vi "Main.vi"(11 "Module Admin":refnum<class "Delacor_lib_QMH_Module Admin.lvclass">) -> ()   [LabVIEW 2019, in "Settings Editor.lvlib"]
doc: "This template is based off of the Queued Message Handler design pattern and the Queued Message Handler project template that ships with LabVIEW.\n\nThe main difference is that the queue is private to this module and communication between modules is performed via Broadcast and Request events.\n\nRequest events are wrapped in public API methods and are handled in the Event Handling Loop (EHL) of this VI. Any module can register for Broadcast events sent by this module. The EHL generates messages based on user interface actions.\n\nThe Message Handling Loop (MHL) processes messages generated by the EHL, or by other messages. The messages are string values, so new messages can be added easily to the Message Cases case structure in the MHL. Each message cluster can also provide an optional value for Message Data, which is a variant that can be converted to whatever message-specific data is required.\n_____\nBased on Delacor QMH Project Template 4.0.0.47.\n_____\nBased on DQMH Project Template 6.1.0.94.\n\n<b>Note:</b> This VI was modified by the <b>Validate DQMH Module</b> tool to add a call to the Error Reported VI at the end of the 'Exit' MHL frame."
uses:
  Settings Editor.lvlib
  <vilib>/Delacor/Delacor QMH/Libraries/Module Admin_class/Delacor_lib_QMH_Module Admin.lvclass
  Acquisition/Signal Type--enum.ctl
  Acquisition/Calibration Values--cluster.ctl
  CML Shared/EEG Channel Settings.ctl
  Module Data--cluster.ctl
  Settings--cluster.ctl
  Settings UI Controls.ctl
  Stop Argument--cluster.ctl
  <vilib>/Delacor/Delacor QMH/Libraries/Message Queue_class/Delacor_lib_QMH_Message Queue.lvclass/Delacor_lib_QMH_Message Queue.ctl
  Update Application Settings Argument--cluster.ctl
  Update Application Settings (Reply Payload)--cluster.ctl
  <vilib>/Delacor/Delacor QMH/Libraries/Module Admin_class/Delacor_lib_QMH_Module Admin.lvclass/Delacor_lib_QMH_Module Admin.ctl
  Set CNV Montage Argument--cluster.ctl
  Set Eyes OC Montage Argument--cluster.ctl
  <vilib>/Utility/sysdir.llb/System Directory Type.ctl
  <vilib>/Delacor/Delacor QMH/Libraries/Message Queue_class/Delacor_lib_QMH_Enqueue Message (Single).vi
  <vilib>/Delacor/Delacor QMH/Libraries/Module Admin_class/Delacor_lib_QMH_Get External Launch.vi
  <vilib>/Utility/error.llb/Error Cluster From Error Code.vi
  <vilib>/ErrorRing/Error Ring.xnode
  <vilib>/Delacor/Delacor QMH/Libraries/Message Queue_class/Delacor_lib_QMH_Message Queue.lvclass
  Acquisition/Acquisition.lvlib
  CML Shared/CML Shared.lvlib
  <vilib>/Utility/miscctls.llb/LVPointTypeDef.ctl
panel:
  in  "Settings.EEG Channels 3":T1={"16 EEG Channels"=[], "Gain"=24} {"16 EEG Channels"."Channel No" step=1}
  in  "Settings.EEG Channels 2":T1={"16 EEG Channels"=[], "Gain"=24} {"16 EEG Channels"."Channel No" step=1}
  in  "Settings Tab":enum32{"Main", "Montage Adder"}(tab)
  in  "Delete Montage":bool
  in  "LSL En enum":enum16{"LSL Disabled", "LSL Enabled"}(ring)
  in  "Log File Base Path":path
  in  "OK":bool
  in  "Cancel":bool
  in  "Soft Trig enum":T2(ring)
  in  "Montages":i32(listbox)
  in  "Add Montage":bool
  out "Name Ch 17":string="Fp1"
  out "En ch 17":bool=TRUE
  out "Ref ch 17":bool
  out "Ref ch 18":bool
  out "Name Ch 18":string="Fp2"
  out "En ch 18":bool=TRUE
  out "Ref ch 19":bool
  out "Name Ch 19":string="F3"
  out "En ch 19":bool=TRUE
  out "Name Ch 20":string="Fz"
  out "En ch 20":bool=TRUE
  out "Ref ch 20":bool
  out "Ref ch 21":bool
  out "Name Ch 21":string="F4"
  out "Ref ch 22":bool
  out "Name Ch 22":string="T3"
  out "Name Ch 23":string="C3"
  out "Ref ch 23":bool
  out "Ref ch 24":bool
  out "Name Ch 24":string="Cz"
  out "Ref ch 25":bool
  out "Name Ch 25":string="C4"
  out "Name Ch 26":string="T4"
  out "Ref ch 26":bool
  out "Ref ch 27":bool
  out "Name Ch 27":string="P3"
  out "Ref ch 28":bool
  out "Name Ch 28":string="Fz"
  out "Ref ch 29":bool
  out "Name Ch 29":string="P4"
  out "En ch 21":bool=TRUE
  out "Ref ch 30":bool
  out "Name Ch 30":string="O1"
  out "En ch 22":bool=TRUE
  out "Ref ch 31":bool
  out "Name Ch 31":string="O2"
  out "En ch 23":bool=TRUE
  out "Ref ch 32":bool=TRUE
  out "Name Ch 32":string="Ref"
  out "En ch 24":bool=TRUE
  out "En ch 25":bool=TRUE
  out "En ch 26":bool=TRUE
  out "En ch 27":bool=TRUE
  out "En ch 28":bool=TRUE
  out "En ch 29":bool=TRUE
  out "En ch 30":bool=TRUE
  out "En ch 31":bool=TRUE
  out "En ch 32":bool
  in  "En ALL":bool
  in  "Name Ch 1":string="Fp1"
  in  "En ch 1":bool=TRUE
  in  "Ref ch 1":bool
  in  "Ref ch 2":bool
  in  "Name Ch 2":string="Fp2"
  in  "En ch 2":bool=TRUE
  in  "Ref ch 3":bool
  in  "Name Ch 3":string="F3"
  in  "En ch 3":bool=TRUE
  in  "Name Ch 4":string="Fz"
  in  "En ch 4":bool=TRUE
  in  "Ref ch 4":bool
  in  "Ref ch 5":bool
  in  "Name Ch 5":string="F4"
  in  "Ref ch 6":bool
  in  "Name Ch 6":string="T3"
  in  "Name Ch 7":string="C3"
  in  "Ref ch 7":bool
  in  "Ref ch 8":bool
  in  "Name Ch 8":string="Cz"
  in  "Ref ch 9":bool
  in  "Name Ch 9":string="C4"
  in  "Name Ch 10":string="T4"
  in  "Ref ch 10":bool
  in  "Ref ch 11":bool
  in  "Name Ch 11":string="P3"
  in  "Ref ch 12":bool
  in  "Name Ch 12":string="Fz"
  in  "Ref ch 13":bool
  in  "Name Ch 13":string="P4"
  in  "En ch 13":bool=TRUE
  in  "Ref ch 14":bool
  in  "Name Ch 14":string="O1"
  in  "En ch 14":bool=TRUE
  in  "Ref ch 15":bool
  in  "Name Ch 15":string="O2"
  in  "En ch 15":bool=TRUE
  in  "Ref ch 16":bool=TRUE
  in  "Name Ch 16":string="Ref"
  in  "En ch 16":bool=TRUE
  in  "En ch 5":bool=TRUE
  in  "En ch 6":bool=TRUE
  in  "En ch 7":bool=TRUE
  in  "En ch 8":bool=TRUE
  in  "En ch 9":bool=TRUE
  in  "En ch 10":bool=TRUE
  in  "En ch 11":bool=TRUE
  in  "En ch 12":bool
  in  "New Montage Name":string
  in  "Save Montage Button":bool
  in  "Cancel Save":bool
  in  "Settings.EEG Channels":T1={"16 EEG Channels"=[], "Gain"=24} {"16 EEG Channels"."Channel No" step=1}
  in  "Calibration Values":T3[](array[typedef])
  in  "Signal Type":T4
  out "error out":errorcluster
  # "Channel 1"
  # "Channel 2"
  # "Channel 3"
  # "Channel 4"
  # "Channel 5"
  # "Channel 6"
  # "Channel 7"
  # "Channel 8"
  # "Channel 9"
  # "Channel 10"
  # "Soft Trigger Settings"
  # "Channel 11"
  # "Channel 12"
  # "LSL Settings"
  # "Channel 13"
  # "Channel 14"
  # "Channel 15"
  # "Channel 16"
  # "Channel 1"
  # "Channel 2"
  # "Channel 3"
  # "Channel 4"
  # "Channel 5"
  # "Channel 6"
  # "Channel 7"
  # "Channel 8"
  # "Channel 9"
  # "Channel 10"
  # "Channel 11"
  # "Channel 12"
  # "Channel 13"
  # "Channel 14"
  # "Channel 15"
  # "Channel 16"
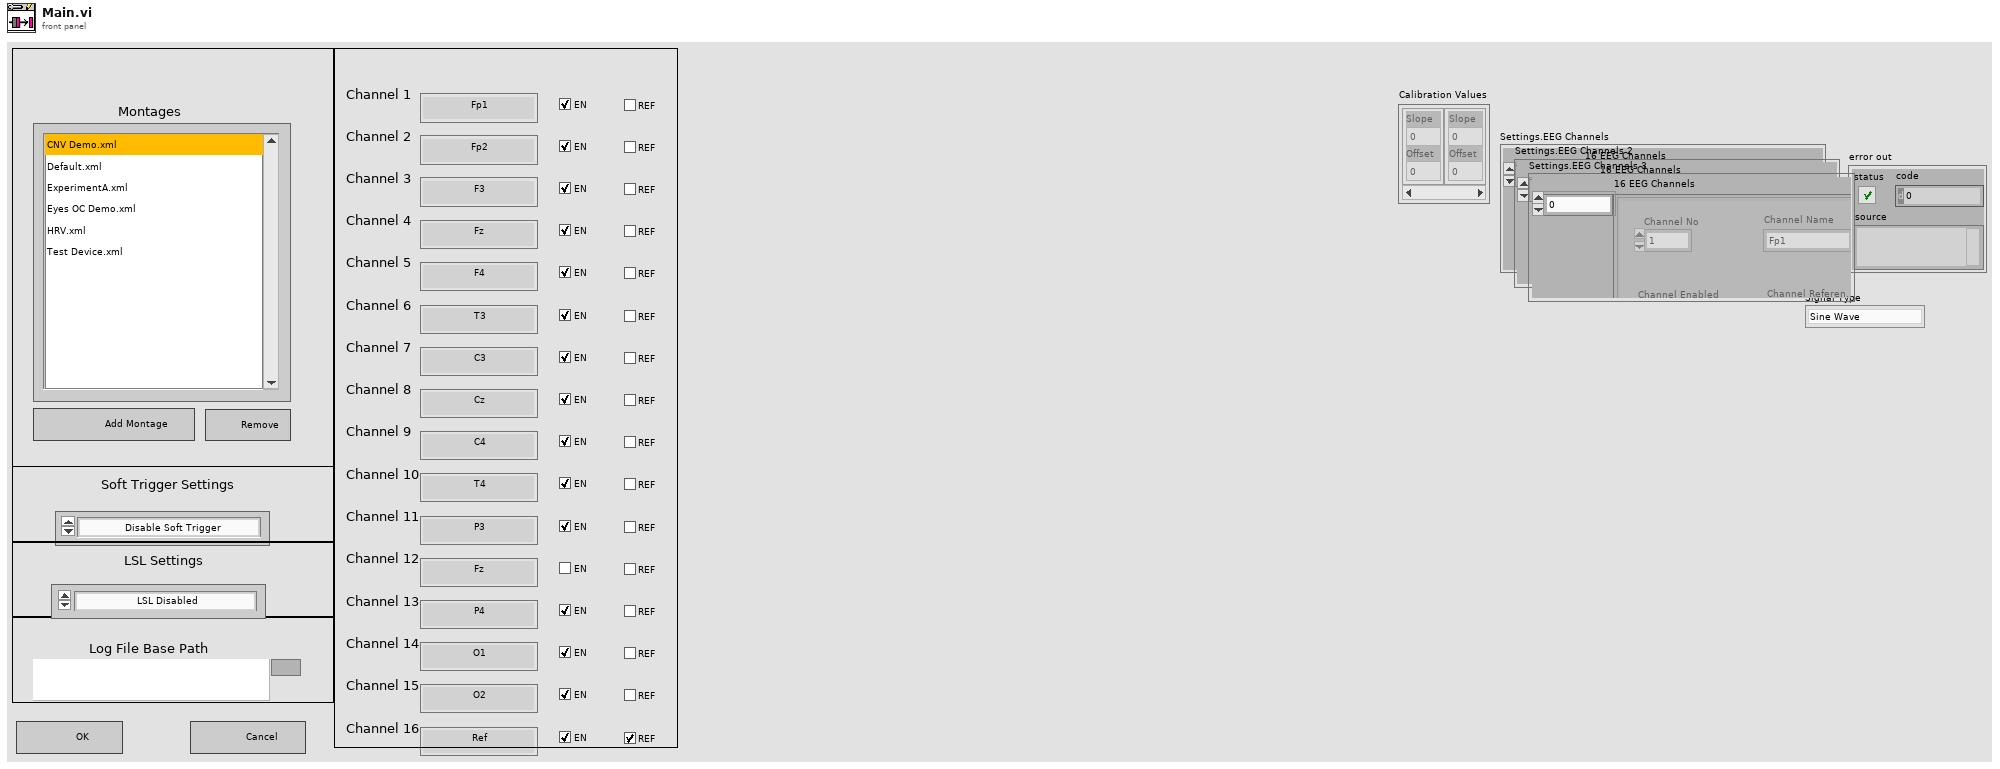
[diagram p1: front panel]
types:
  T1 = typedef "CML Shared.lvlib/EEG Channel Settings.ctl" = cluster{"16 EEG Channels":cluster{"Channel Name":string, "Channel No":u8, "Channel Enabled":bool, "Channel Referenced":bool}[], "Gain":u8}
  T2 = enum16{"Disable Soft Trigger", "Enable Soft Trigger"}
  T3 = typedef "Acquisition.lvlib/Calibration Values--cluster.ctl" = cluster{"Slope":dbl, "Offset":dbl}
  T4 = typedef "Acquisition.lvlib/Signal Type--enum.ctl" = enum16{"Sine Wave", "Square with Noise"}
  T5 = typedef "Settings Editor.lvlib/Request Events--cluster.ctl" = cluster{"Stop Module":refnum<user-event>, "Show Panel":refnum<user-event>, "Hide Panel":refnum<user-event>, "Get Module Execution Status":refnum<user-event>, "Show Diagram":refnum<user-event>, "Update Application Settings":refnum<user-event>, "Set CNV Montage":refnum<user-event>, "Set Eyes OC Montage":refnum<user-event>}
  T6 = typedef "Settings Editor.lvlib/Module Data--cluster.ctl" = cluster{"Settings":T7, "Settings Tab":refnum<vi>, "Controls UI":T8}
  T7 = typedef "Settings Editor.lvlib/Settings--cluster.ctl" = cluster{"Signal Type":T4, "Calibration Array":T3[], "Log File Base Path":path, "EEG Channels":T1, "Soft Trig enum":enum16{"Disable Soft Trigger", "Enable Soft Trigger"}, "Montage selection":cluster{"Montages Ref":refnum<vi>, "Selected Montage Number":u8, "Montages Names":string[]}, "LSL En enum":enum16{"LSL Disabled", "LSL Enabled"}}
  T8 = typedef "Settings Editor.lvlib/Settings UI Controls.ctl" = cluster{"En ch 1":refnum<vi>, "En ch 2":refnum<vi>, "En ch 3":refnum<vi>, "En ch 4":refnum<vi>, "En ch 5":refnum<vi>, "En ch 6":refnum<vi>, "En ch 7":refnum<vi>, "En ch 8":refnum<vi>, "En ch 9":refnum<vi>, "En ch 10":refnum<vi>, "En ch 11":refnum<vi>, "En ch 12":refnum<vi>, "En ch 13":refnum<vi>, "En ch 14":refnum<vi>, "En ch 15":refnum<vi>, "En ch 16":refnum<vi>, "Delete Montage":refnum<vi>}
  T9 = enum32{"invalid lock state", "Not Locked", "Locked (No Password)", "Password-protected"}
  T10 = typedef "Settings Editor.lvlib/Stop Argument--cluster.ctl" = cluster{"Origin":string, "Exit via Stop Module Req?":bool, "Wait for Module to stop?":bool}
  T11 = typedef "Settings Editor.lvlib/Update Application Settings Argument--cluster.ctl" = cluster{"Wait Notifier":refnum<notifier>, "wait for reply":bool}
  T12 = typedef "Settings Editor.lvlib/Set CNV Montage Argument--cluster.ctl" = cluster{"Boolean":bool}
  T13 = typedef "Settings Editor.lvlib/Set Eyes OC Montage Argument--cluster.ctl" = cluster{"Boolean":bool}
  T14 = enum32{"Invalid", "Standard", "Closed", "Hidden", "Minimized", "Maximized"}
  T15 = typedef "LVPointTypeDef.ctl" = cluster{"Horizontal":i16, "Vertical":i16}
  T16 = typedef "Settings Editor.lvlib/Update Application Settings (Reply Payload)--cluster.ctl" = cluster{"Settings":T7, "error":errorcluster}
  T17 = typedef "System Directory Type.ctl" = i32
  T18 = cluster{"Channel Name":string, "Channel No":u8, "Channel Enabled":bool, "Channel Referenced":bool}[]
  T19 = cluster{"Channel Name":string, "Channel No":u8, "Channel Enabled":bool, "Channel Referenced":bool}
  T20 = cluster{"Montages Ref":refnum<vi>, "Selected Montage Number":u8, "Montages Names":string[]}
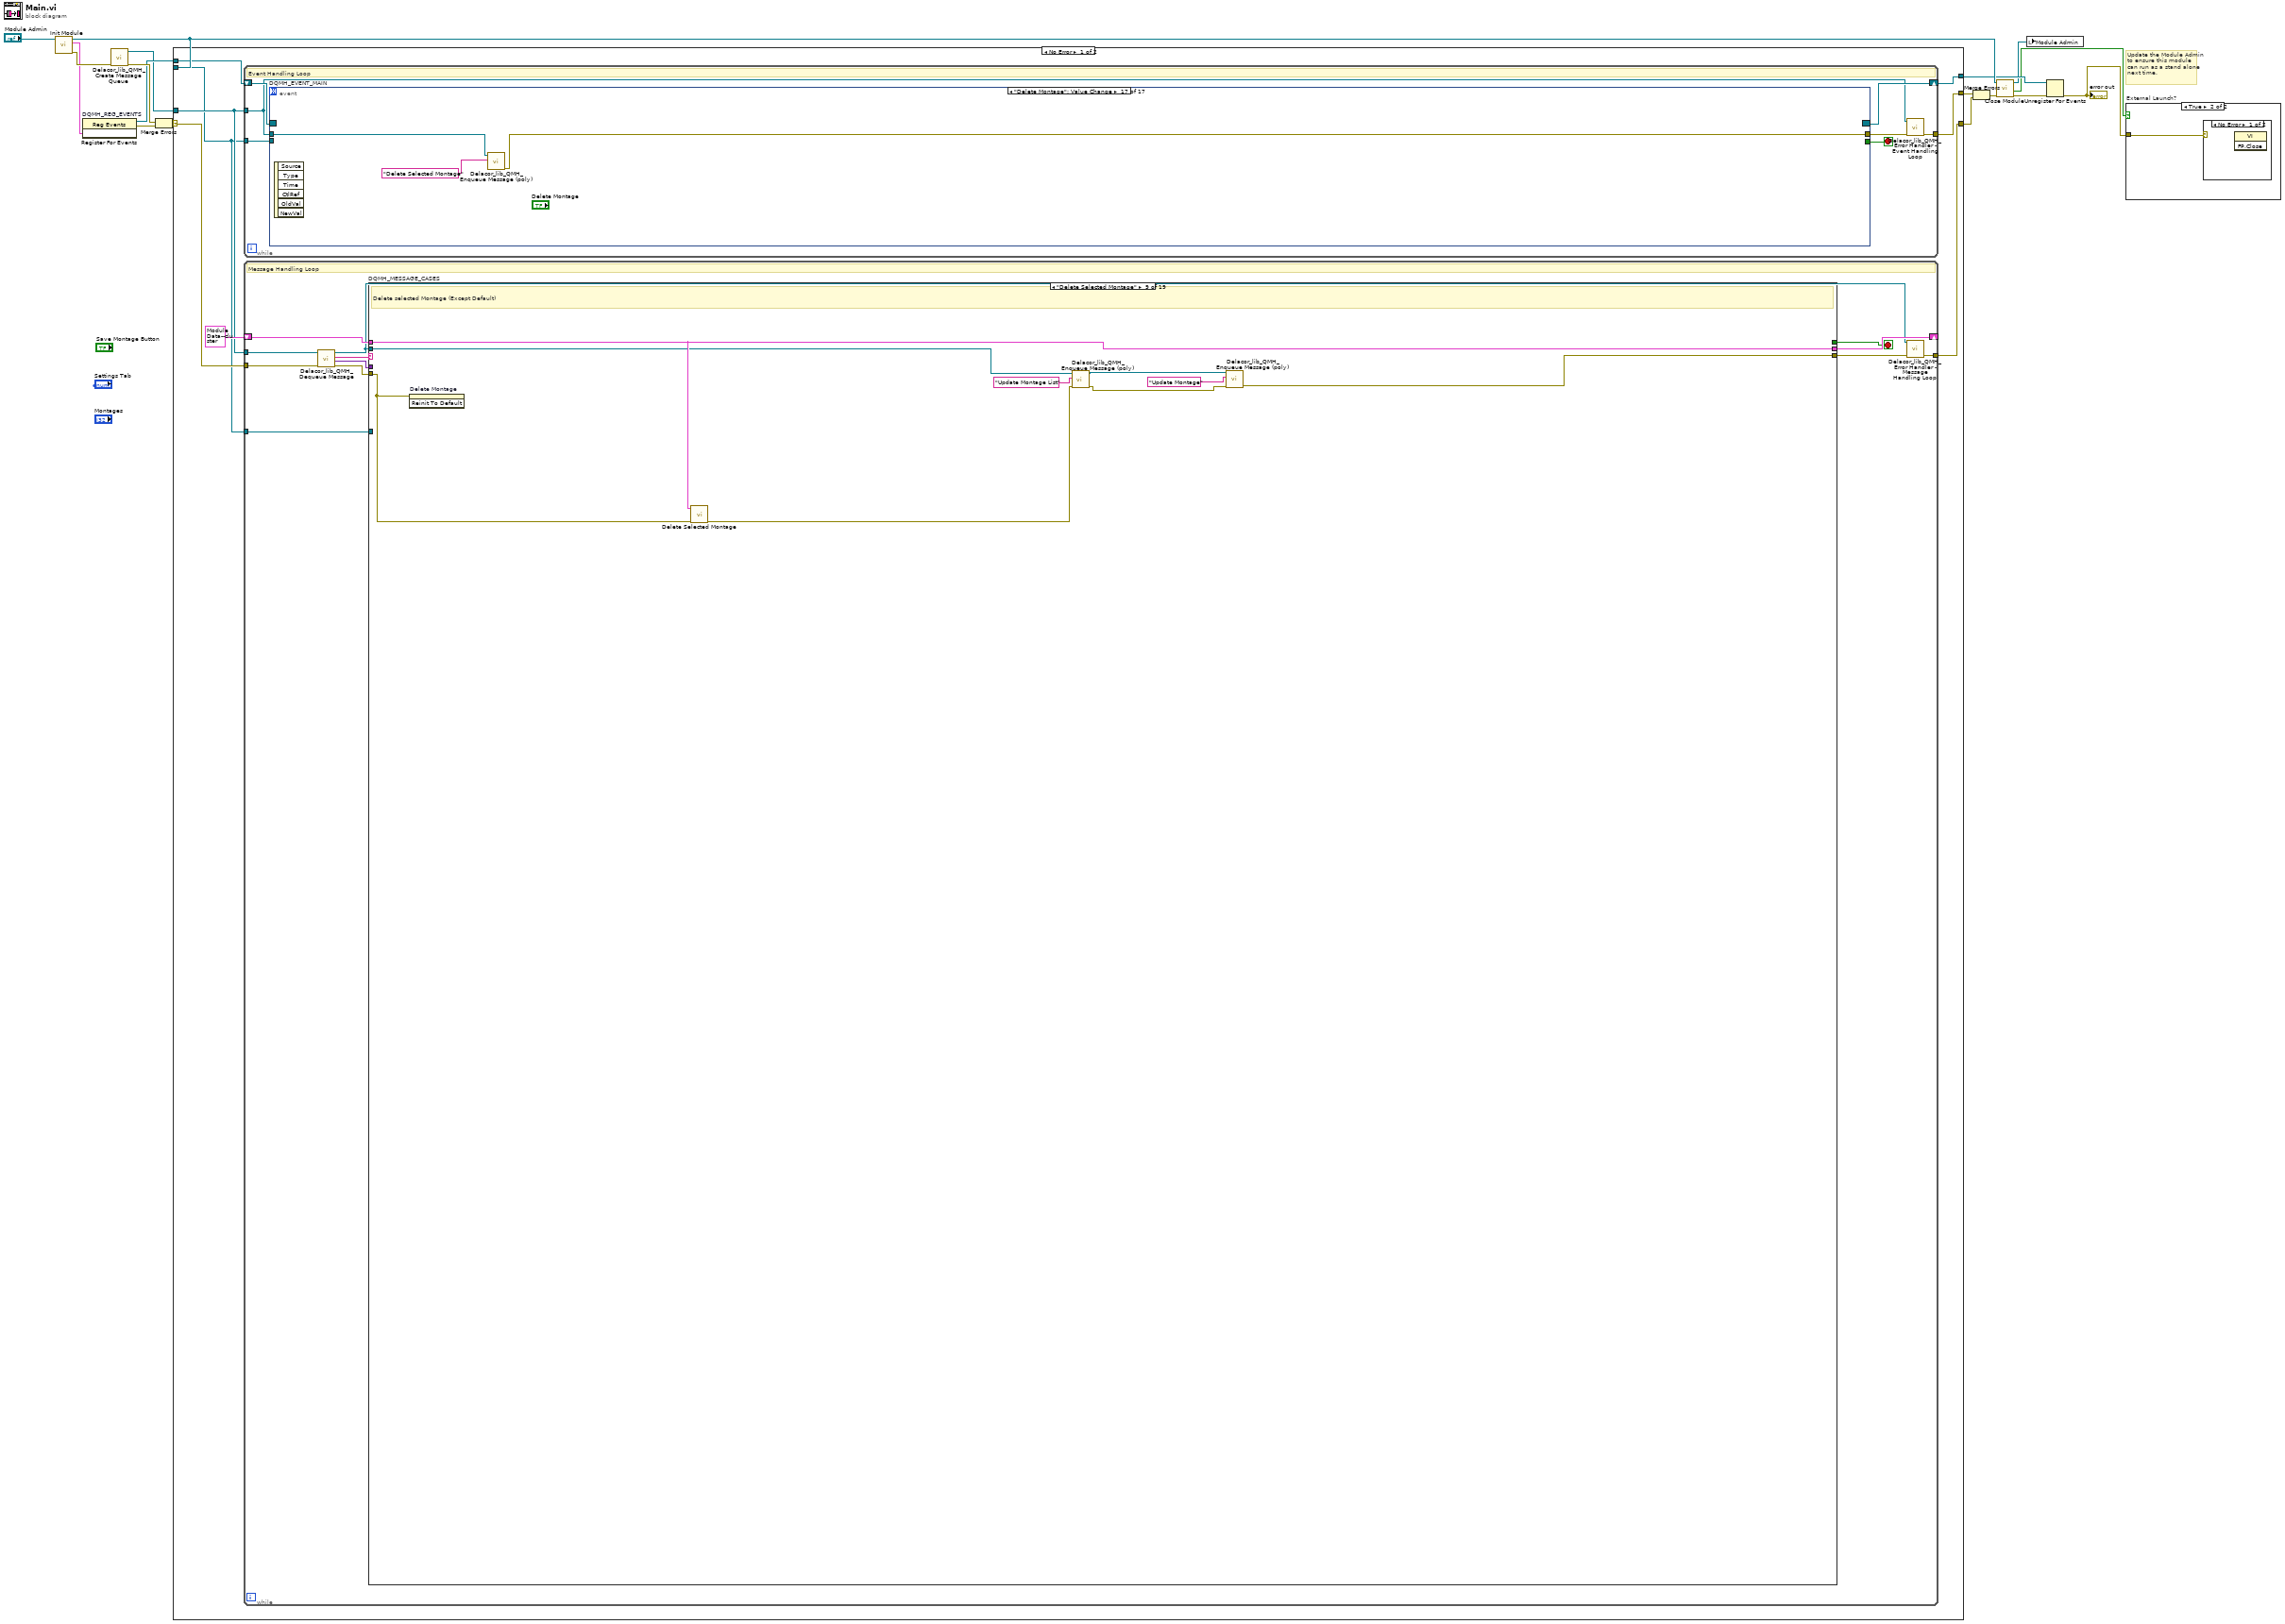
[diagram p0: block diagram]
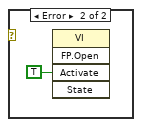
[diagram p3: hidden frame]
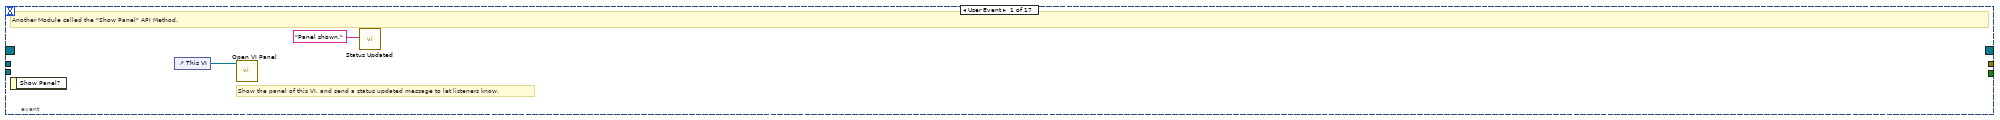
[diagram p4: hidden frame]
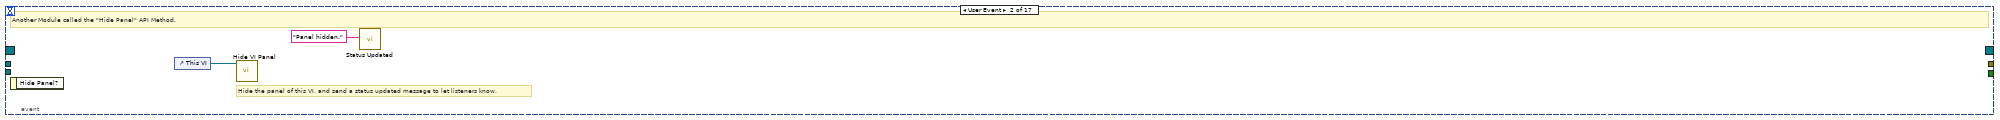
[diagram p5: hidden frame]
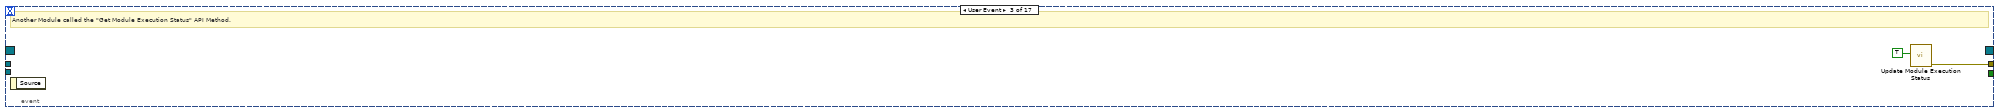
[diagram p6: hidden frame]
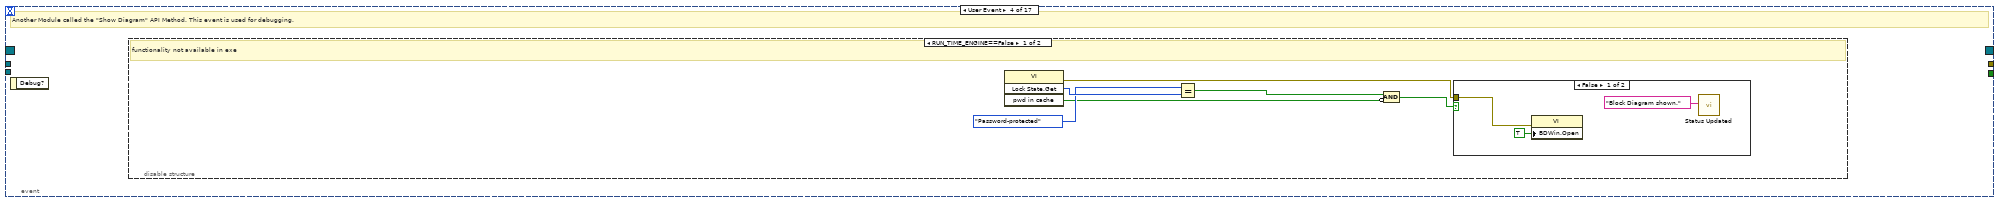
[diagram p7: hidden frame]
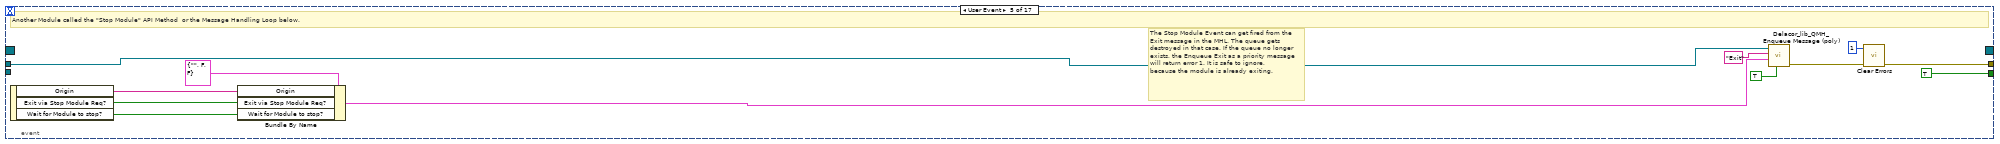
[diagram p10: hidden frame]
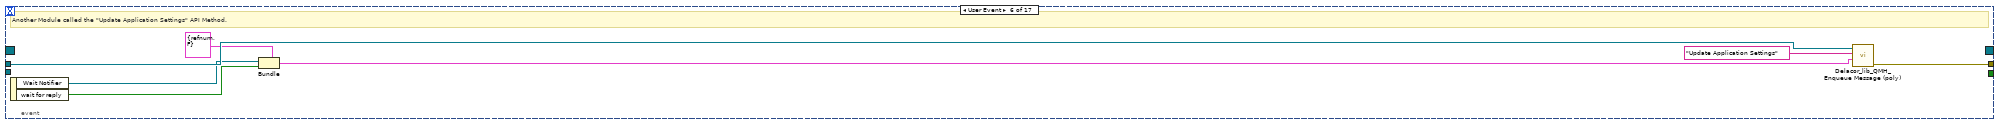
[diagram p11: hidden frame]
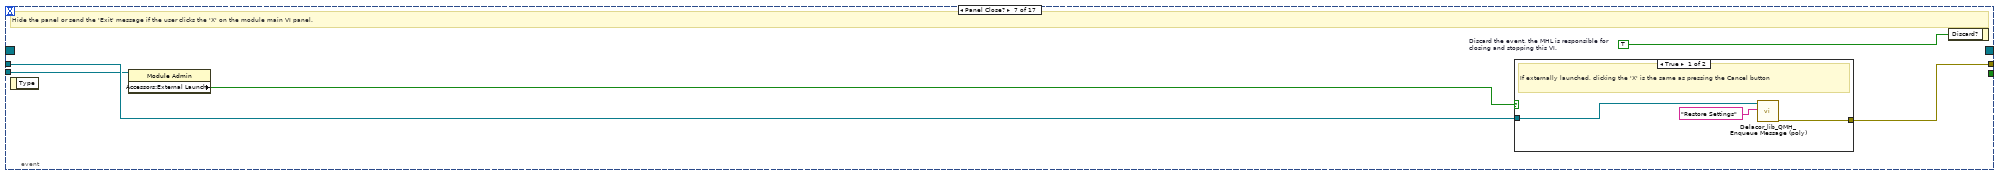
[diagram p12: hidden frame]
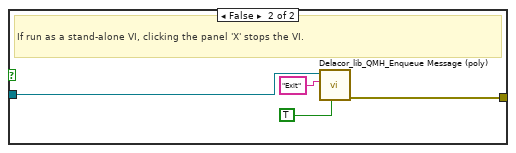
[diagram p13: hidden frame]
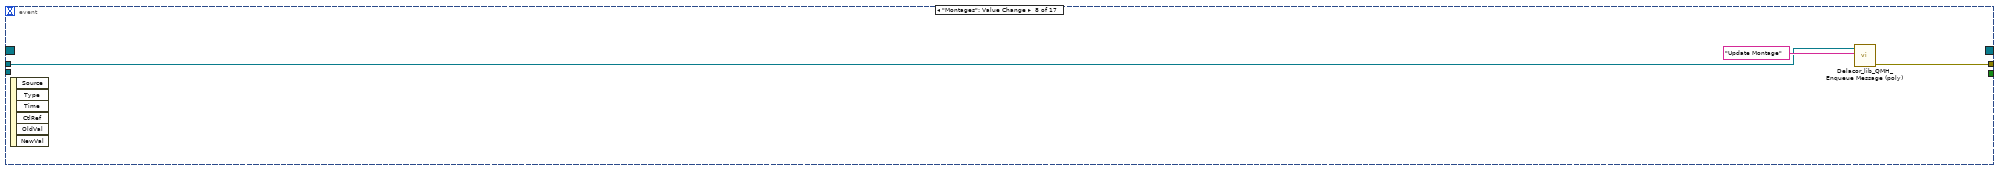
[diagram p14: hidden frame]
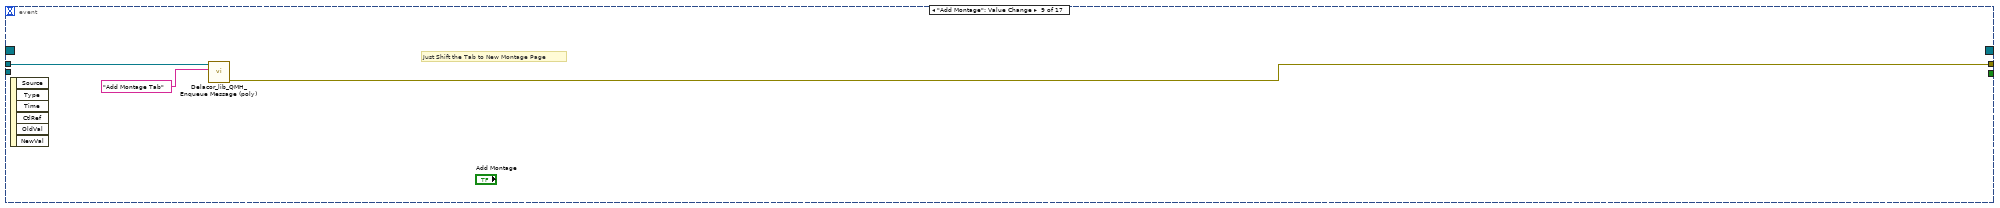
[diagram p15: hidden frame]
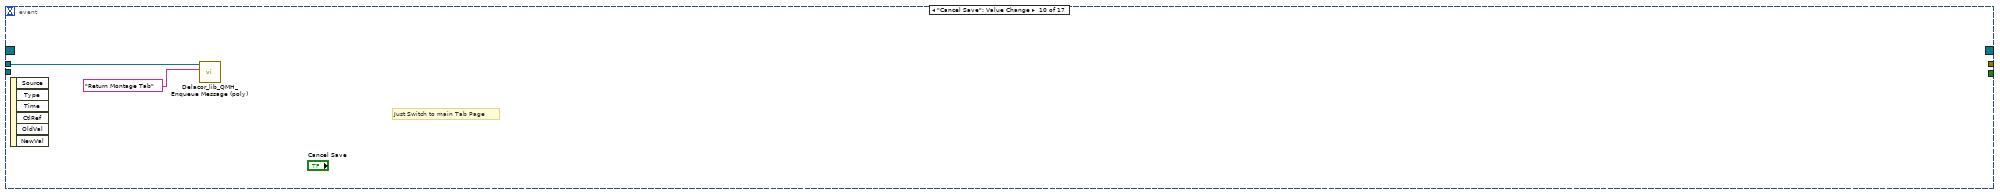
[diagram p16: hidden frame]
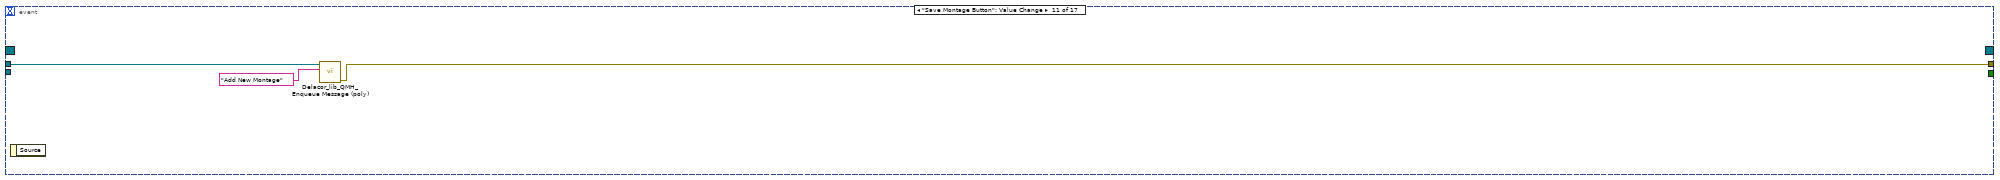
[diagram p17: hidden frame]
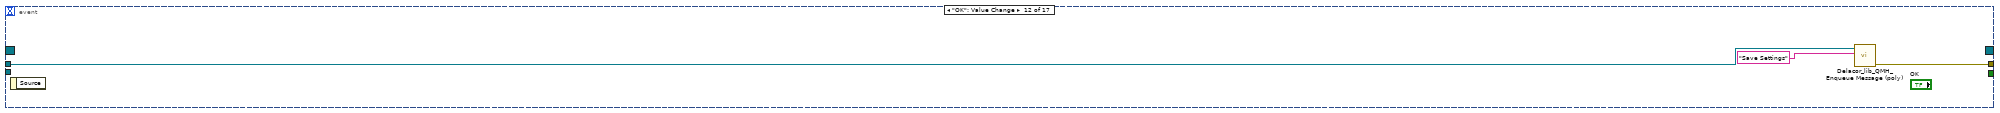
[diagram p18: hidden frame]
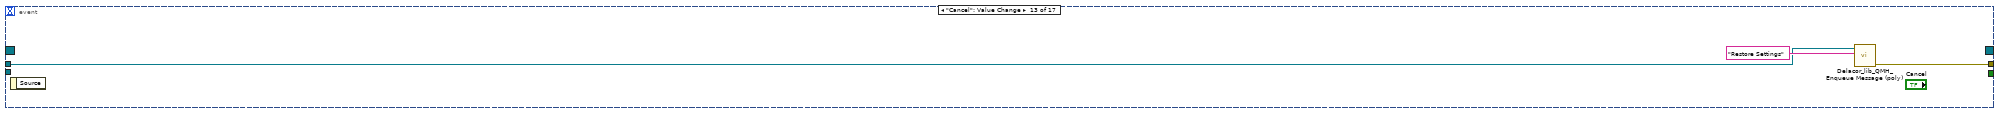
[diagram p19: hidden frame]
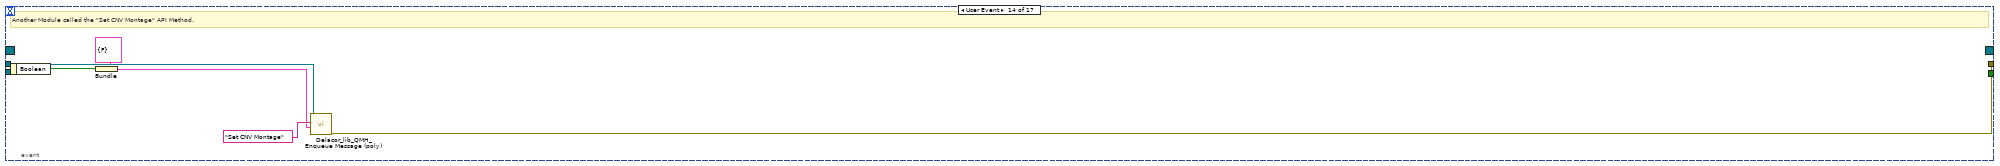
[diagram p20: hidden frame]
diagram:
  # "Update the Module Admin to ensure this module can run as a stand alone next time."
  n1 = call "Init Module.vi"("Singleton Module Admin in"="Module Admin") -> ("error out"=w16:errorcluster, "Settings Editor Request Events"=w5:T5, "Singleton Module Admin out"=w8:refnum<class "Delacor_lib_QMH_Module Admin.lvclass">)  [unwired: 8 in]
  n2 = register-events "DQMH_REG_EVENTS"(w5) -> (reference out=w6:refnum<event-registration>, error out=w9:errorcluster)  [unwired: 2 in]
  n3 = call <vilib>:"Delacor_lib_QMH_Create Message Queue.vi"("error in"=w16) -> ("error out"=w11:errorcluster, "Message Queue"=w4:refnum<class "Delacor_lib_QMH_Message Queue.lvclass">)  [unwired: 9 in]
  n4 = Merge Errors(w11, w9) -> (w10:errorcluster)
  n5 = case shown="No Error" w10 {
    selector: w10 -> [w23 w909]
    tunnel: [w25 w908] -> w17
    tunnel: [w22 w915] -> w7
    tunnel: w6 -> [w20 w915]
    tunnel: w4 -> [w19 w910]
    tunnel: [w24 _] -> w14
    tunnel: w8 -> [w18 w911]
    frame No Error {
      n6 = while {
        tunnel: w19 -> [w26]
        shift-right: [w29] -> w22
        shift-left: w20 -> [w30]
        tunnel: [w31] -> w24
        tunnel: w18 -> [w27]
        stop <- w28 stop-if-true
        # "Event Handling Loop"
        n7 = event "DQMH_EVENT_MAIN" shown="[16] \"Delete Montage\": Value Change" {
          selector: w30 -> [_ _ _ _ _ _ _ _ _ _ _ _ _ _ _ _ _]
          dyn-events: [_ _ _ _ _ _ _ _ _ _ _ _ _ _ _ _ _] -> w29
          timeout: _ -> [_ _ _ _ _ _ _ _ _ _ _ _ _ _ _ _ _]
          tunnel: [_ _ _ _ TRUE ("Discard?") _ _ _ _ _ _ _ _ _ _ _ _] -> w28
          tunnel: w26 -> [_ _ _ _ w55 w66 w69 w80 w83 w85 w88 w90 w94 w101 w107 w110 w113]
          tunnel: [_ _ w38 _ w58 w62 w71 w79 w82 _ w87 w91 w93 w96 w102 w108 w112] -> w32
          tunnel: w27 -> [_ _ _ _ _ _ w68 _ _ _ _ _ _ _ _ _ _]
          event User Event {
            # "Show the panel of this VI, and send a status updated message to let listeners know."
            # "Another Module called the \"Show Panel\" API Method."
            n8 = event-data() -> ()  [unwired: 1 in, 1 out]
            n9 = control-ref of="This VI"() -> (w34:refnum<vi>)
            n10 = call "Open VI Panel.vi"("VI"=w34) -> ()  [unwired: 10 in, 1 out]
            n11 = call "Status Updated.vi"("Status"="Panel shown." ("format string")) -> ()  [unwired: 10 in, 1 out]
          }
          event User Event {
            # "Hide the panel of this VI, and send a status updated message to let listeners know."
            # "Another Module called the \"Hide Panel\" API Method."
            n12 = event-data() -> ()  [unwired: 1 in, 1 out]
            n13 = control-ref of="This VI"() -> (w36:refnum<vi>)
            n14 = call "Hide VI Panel.vi"("VI"=w36) -> ()  [unwired: 10 in, 1 out]
            n15 = call "Status Updated.vi"("Status"="Panel hidden." ("format string")) -> ()  [unwired: 10 in, 1 out]
          }
          event User Event {
            # "Another Module called the \"Get Module Execution Status\" API Method."
            n16 = event-data() -> ()  [unwired: 1 in, 1 out]
            n17 = call "Update Module Execution Status.vi"("Running?"=TRUE) -> ("error out"=w38:errorcluster)  [unwired: 10 in]
          }
          event User Event {
            # "Another Module called the \"Show Diagram\" API Method. This event is used for debugging."
            n18 = event-data() -> ()  [unwired: 1 in, 1 out]
            n19 = disable-structure shown="RUN_TIME_ENGINE==False" {
              frame condition #0 (active) {
                # "functionality not available in exe"
                n20 = invoke class="VI" method="Lock State.Get"() -> (error out=w44:errorcluster, "Get Lock State"=w43:T9, "pwd in cache"=w40:bool)  [unwired: 4 in, 1 out]
                n21 = Equal?(x=T9."Password-protected", y=w43) -> (x = y?=w41:bool)
                n22 = Compound Arithmetic op=AND(w41, invert w40) -> (w39:bool)
                n23 = case shown="False" w39 {
                  tunnel: w44 -> [w47 _]
                  frame False {
                    n24 = property class="VI"(error in=w47, "BDWin.Open"=TRUE ("Block Diagram Window:Open")) -> ()  [unwired: 1 in, 2 out]
                    n25 = call "Status Updated.vi"("Status"="Block Diagram shown." ("format string")) -> ()  [unwired: 10 in, 1 out]
                  }
                  frame True {
                    # "Password-protected VI, and the password is not in the cache. Do not show the diagram."
                  }
                }
              }
              frame condition #1 {
              }
            }
          }
          event User Event {
            # "The Stop Module Event can get fired from the Exit message in the MHL. The queue gets destroyed in that case. If the queue no longer exists, the Enqueue Exit as a priority message will return error 1. It is safe to ignore, because the module is already exiting."
            # "Another Module called the \"Stop Module\" API Method  or the Message Handling Loop below."
            n26 = event-data() -> ("Origin"=w48:string, "Exit via Stop Module Req?"=w51:bool, "Wait for Module to stop?"=w50:bool)  [unwired: 1 in]
            n27 = Bundle By Name(cluster=T10 {"Origin"="", "Exit via Stop Module Req?"=FALSE, "Wait for Module to stop?"=FALSE} ("Stop Argument"), "Origin"=w48, "Exit via Stop Module Req?"=w51, "Wait for Module to stop?"=w50) -> (w49:T10)
            n28 = call-poly <vilib>:"Delacor_lib_QMH_Enqueue Message (poly).vi"("Priority Message? (F)"=TRUE, "Message Data"=w49, "Message"="Exit", "Message Queue in"=w55) -> ("error out"=w59:errorcluster)  [unwired: 6 in, 1 out]
            n29 = call <vilib>:"Clear Errors.vi"("error in (no error)"=w59, "specific error code to clear (0: all)"=1) -> ("error out"=w58:errorcluster)  [unwired: 4 in, 1 out]
          }
          event User Event {
            # "Another Module called the \"Update Application Settings\" API Method."
            n30 = event-data() -> ("Wait Notifier"=w61:refnum<notifier>, "wait for reply"=w60:bool)  [unwired: 1 in]
            n31 = Bundle(cluster=T11 {"Wait Notifier"=refnum, "wait for reply"=FALSE} ("Update Application Settings Argument"), "Wait Notifier"=w61, "wait for reply"=w60) -> (w63:T11)
            n32 = call-poly <vilib>:"Delacor_lib_QMH_Enqueue Message (poly).vi"("Message Data"=w63, "Message"="Update Application Settings", "Message Queue in"=w66) -> ("error out"=w62:errorcluster)  [unwired: 7 in, 1 out]
          }
          event Panel Close? {
            w70 = TRUE  # Discard the event, the MHL is responsible for closing and stopping this VI.
            # "Hide the panel or send the 'Exit' message if the user clicks the 'X' on the module main VI panel."
            n33 = event-data() -> ()  [unwired: 1 in, 1 out]
            n34 = property class="Module Admin"(reference=w68) -> ("Accessors:External Launch"=w67:bool)  [unwired: 1 in, 2 out]
            n35 = case shown="True" w67 {
              tunnel: w69 -> [w73 w77]
              tunnel: [w72 w78] -> w71
              frame True {
                # "If externally launched, clicking the 'X' is the same as pressing the Cancel button"
                n36 = call-poly <vilib>:"Delacor_lib_QMH_Enqueue Message (poly).vi"("Message"="Restore Settings", "Message Queue in"=w73) -> ("error out"=w72:errorcluster)  [unwired: 8 in, 1 out]
              }
              frame False {
                # "If run as a stand-alone VI, clicking the panel 'X' stops the VI."
                n37 = call-poly <vilib>:"Delacor_lib_QMH_Enqueue Message (poly).vi"("Priority Message? (F)"=TRUE, "Message"="Exit", "Message Queue in"=w77) -> ("error out"=w78:errorcluster)  [unwired: 7 in, 1 out]
              }
            }
            n38 = event-data("Discard?"=w70) -> ()  [unwired: 1 in, 1 out]
          }
          event "Montages": Value Change {
            n39 = event-data() -> ()  [unwired: 1 in, 6 out]
            n40 = call-poly <vilib>:"Delacor_lib_QMH_Enqueue Message (poly).vi"("Message"="Update Montage", "Message Queue in"=w80) -> ("error out"=w79:errorcluster)  [unwired: 8 in, 1 out]
          }
          event "Add Montage": Value Change {
            # "Just Shift the Tab to New Montage Page"
            n41 = event-data() -> ()  [unwired: 1 in, 6 out]
            n42 = call-poly <vilib>:"Delacor_lib_QMH_Enqueue Message (poly).vi"("Message"="Add Montage Tab", "Message Queue in"=w83) -> ("error out"=w82:errorcluster)  [unwired: 8 in, 1 out]
          }
          event "Cancel Save": Value Change {
            # "Just Switch to main Tab Page"
            n43 = event-data() -> ()  [unwired: 1 in, 6 out]
            n44 = call-poly <vilib>:"Delacor_lib_QMH_Enqueue Message (poly).vi"("Message"="Return Montage Tab", "Message Queue in"=w85) -> ()  [unwired: 8 in, 2 out]
          }
          event "Save Montage Button": Value Change {
            n45 = event-data() -> ()  [unwired: 1 in, 1 out]
            n46 = call-poly <vilib>:"Delacor_lib_QMH_Enqueue Message (poly).vi"("Message"="Add New Montage", "Message Queue in"=w88) -> ("error out"=w87:errorcluster)  [unwired: 8 in, 1 out]
          }
          event "OK": Value Change {
            n47 = event-data() -> ()  [unwired: 1 in, 1 out]
            n48 = call-poly <vilib>:"Delacor_lib_QMH_Enqueue Message (poly).vi"("Message"="Save Settings", "Message Queue in"=w90) -> ("error out"=w91:errorcluster)  [unwired: 8 in, 1 out]
          }
          event "Cancel": Value Change {
            n49 = event-data() -> ()  [unwired: 1 in, 1 out]
            n50 = call-poly <vilib>:"Delacor_lib_QMH_Enqueue Message (poly).vi"("Message"="Restore Settings", "Message Queue in"=w94) -> ("error out"=w93:errorcluster)  [unwired: 8 in, 1 out]
          }
          event User Event {
            # "Another Module called the \"Set CNV Montage\" API Method."
            n51 = event-data() -> ("Boolean"=w97:bool)  [unwired: 1 in]
            n52 = Bundle(cluster=T12 {"Boolean"=FALSE} ("Set CNV Montage Argument"), "Boolean"=w97) -> (w98:T12)
            n53 = call-poly <vilib>:"Delacor_lib_QMH_Enqueue Message (poly).vi"("Message Data"=w98, "Message"="Set CNV Montage", "Message Queue in"=w101) -> ("error out"=w96:errorcluster)  [unwired: 7 in, 1 out]
          }
          event User Event {
            # "Another Module called the \"Set Eyes OC Montage\" API Method."
            n54 = event-data() -> ("Boolean"=w103:bool)  [unwired: 1 in]
            n55 = Bundle(cluster=T13 {"Boolean"=FALSE} ("Set Eyes OC Montage Argument"), "Boolean"=w103) -> (w104:T13)
            n56 = call-poly <vilib>:"Delacor_lib_QMH_Enqueue Message (poly).vi"("Message Data"=w104, "Message"="Set Eyes OC Montage", "Message Queue in"=w107) -> ("error out"=w102:errorcluster)  [unwired: 7 in, 1 out]
          }
          event "En ALL": Value Change {
            n57 = event-data() -> ("NewVal"=w109:bool)  [unwired: 1 in, 2 out]
            n58 = call-poly <vilib>:"Delacor_lib_QMH_Enqueue Message (poly).vi"("Message Data"=w109, "Message"="Enable all Ch settings", "Message Queue in"=w110) -> ("error out"=w108:errorcluster)  [unwired: 7 in, 1 out]
          }
          event "Delete Montage": Value Change {
            n59 = event-data() -> ()  [unwired: 1 in, 6 out]
            n60 = call-poly <vilib>:"Delacor_lib_QMH_Enqueue Message (poly).vi"("Message"="Delete Selected Montage", "Message Queue in"=w113) -> ("error out"=w112:errorcluster)  [unwired: 8 in, 1 out]
          }
        }
        n61 = call-dynamic "Delacor_lib_QMH_Error Handler - Event Handling Loop.vi"("error in"=w32, "Message Queue in"=w26) -> ("dup error in"=w31:errorcluster)  [unwired: 8 in, 1 out]
      }
      n62 = while {
        tunnel: w19 -> [w118]
        shift-right: [w121] -> _
        shift-left: T6 {"Settings"={"Signal Type"=enum."Sine Wave", "Calibration Array"=[{"Slope"=1.0, "Offset"=0.0}], "Log File Base Path"=path "", "EEG Channels"={"16 EEG Channels"=[], "Gain"=24}, "Soft Trig enum"=enum."Disable Soft Trigger", "Montage selection"={"Montages Ref"=refnum, "Selected Montage Number"=0, "Montages Names"=[]}, "LSL En enum"=enum."LSL Disabled"}, "Settings Tab"=refnum, "Controls UI"={"En ch 1"=refnum, "En ch 2"=refnum, "En ch 3"=refnum, "En ch 4"=refnum, "En ch 5"=refnum, "En ch 6"=refnum, "En ch 7"=refnum, "En ch 8"=refnum, "En ch 9"=refnum, "En ch 10"=refnum, "En ch 11"=refnum, "En ch 12"=refnum, "En ch 13"=refnum, "En ch 14"=refnum, "En ch 15"=refnum, "En ch 16"=refnum, "Delete Montage"=refnum}} ("Data Cluster") -> [w122]
        tunnel: w23 -> [w125]
        tunnel: [w123] -> w25
        tunnel: w18 -> [w116]
        stop <- w120 stop-if-true
        # "Message Handling Loop"
        n63 = call-dynamic "Delacor_lib_QMH_Dequeue Message.vi"("error in"=w125, "Message Queue in"=w118) -> ("error out"=w124:errorcluster, "Message Data"=w119:variant, "Message"=w115:string, "Message Queue out"=w117:refnum<class "Delacor_lib_QMH_Message Queue.lvclass">)  [unwired: 6 in]
        n64 = case "DQMH_MESSAGE_CASES" shown="\"Delete Selected Montage\"" w115 {
          selector: w115 -> [_ _ _ _ _ _ _ _ _ _ _ _ _ _ _ _ _ _ w895]
          tunnel: w117 -> [w158 _ _ _ w397 w520 _ _ w657 _ _ _ _ w702 _ _ w865 w887 _]
          tunnel: w124 -> [w154 w255 w271 w385 w396 w519 w647 w650 w651 w682 w690 w695 w700 w791 w860 w862 w872 w893 w897]
          tunnel: [w153 w255 w272 w386 w508 w631 w647 w649 w652 w660 w689 w694 w699 w790 w859 w862 w868 w890 w898] -> w126
          tunnel: w122 -> [w242 w254 w265 w276 w468 w591 w646 w648 w659 w679 w683 w693 w698 w789 w792 w861 w867 w886 w896]
          tunnel: [w144 w254 w265 w392 w512 w635 w646 w648 w659 w679 w683 w693 w698 w789 w792 w861 w867 w886 w896] -> w121
          tunnel: [_ _ _ _ _ _ _ _ _ _ _ _ _ _ _ _ _ w885 _] -> w120
          tunnel: w119 -> [_ _ w270 _ _ _ _ _ _ w681 _ _ _ _ _ _ w866 w884 _]
          tunnel: w116 -> [w243 _ _ _ _ _ _ _ _ _ _ _ _ _ _ _ w864 w879 _]
          frame "Initialize" {
            w148 = T17 2 items=["User Home"=0, "User Desktop"=1, "User Documents"=2, "User Application Data"=3, "User Preferences"=4, "User Temporary"=5, "Public Documents"=6, "Public Application Data"=7, "Public Preferences"=8, "Public Cache"=13, "System Core Libraries"=9, "System Installed Libraries"=10, "Application Files"=11, "Boot Volume Root"=12] ("system directory type")
            # "Initialize - Any operation that needs to be done before the module can receive messages. Synchronize Caller Events.vi will inform Start Module.vi that the module has launched and is ready to receive messages. Module Did Init.vi will broadcast that the module initialized."
            n65 = call "Load Settings from XML.vi"() -> ("Settings out"=w166:T7)  [unwired: 10 in, 1 out]
            n66 = control-ref of="Settings Tab"() -> (w157:refnum<vi>)
            n67 = disable-structure shown="Enabled" {
              frame Disabled {
                n68 = property on="Pane" class="Pane"("Origin"=T15 {"Horizontal"=0, "Vertical"=0}) -> ()  [unwired: 2 in, 2 out]
              }
              frame Enabled {
              }
            }
            n69 = call "Synchronize Caller Events.vi"("error in (no error)"=w154, "Singleton Module Admin in"=w243) -> ("error out"=w251:errorcluster, "Singleton Module Admin out"=w239:refnum<class "Delacor_lib_QMH_Module Admin.lvclass">)  [unwired: 8 in]
            n70 = property class="Module Admin"(reference=w239) -> ("Accessors:External Launch"=w247:bool)  [unwired: 1 in, 2 out]
            n71 = Unbundle By Name(w166) -> ("Soft Trig enum"=w167:T2, "LSL En enum"=w146:enum16{"LSL Disabled", "LSL Enabled"})
            n72 = call "Module Name--constant.vi"() -> ("Module Name"=w240:string)  [unwired: 11 in]
            n73 = Bundle By Name(cluster=w242, "Settings"=w166, "Settings Tab"=w157) -> (w163:T6)
            n74 = Unbundle(w166) -> ("Log File Base Path"=w152:path, "EEG Channels"=w234:T1)  [unwired: 5 out]
            n75 = call "Module Did Init.vi"("error in (no error)"=w251, "Initialized?"=TRUE, "Origin"=w240) -> ("error out"=w153:errorcluster)  [unwired: 8 in]
            n76 = local write "Soft Trig enum"(w167) -> ()
            n77 = local write "LSL En enum"(w146) -> ()
            n78 = call "Module Name--constant.vi"() -> ("Module Name"=w250:string)  [unwired: 11 in]
            n79 = local write "Log File Base Path"(w152) -> ()
            n80 = Unbundle By Name(w234) -> ("16 EEG Channels"=w233:T18)
            n81 = Select(t=T14."Hidden" ("State"), s=w247, f=T14."Standard" ("State")) -> (s? t:f=w244:T14)
            n82 = property class="VI"("Front Panel.Title"=w250) -> (reference out=w249:refnum<vi>, error out=w238:errorcluster)  [unwired: 2 in]
            n83 = invoke class="VI" method="FP.Open"(reference=w249, error in=w238, "State"=w244) -> (reference out=w248:refnum<vi>, error out=w252:errorcluster)  [unwired: 2 in, 3 out]
            n84 = call <vilib>:"Get System Directory.vi"("system directory type"=w148) -> ("system directory"=w147:path)  [unwired: 10 in]
            n85 = call <vilib>:"Check if File or Folder Exists.vi"("path"=w152) -> ("file or folder exists?"=w151:bool, "dup path"=w150:path)  [unwired: 8 in, 1 out]
            n86 = invoke class="VI" method="FP.Center"(reference=w248, error in=w252) -> ()  [unwired: 1 in, 3 out]
            n87 = call-poly <vilib>:"Delacor_lib_QMH_Enqueue Message (poly).vi"("error in"=w153, "Message"="Update Montage", "Message Queue in"=w158) -> ()  [unwired: 7 in, 2 out]
            n88 = Select(t=w150, s=w151, f=w147) -> (s? t:f=w149:path)
            n89 = call "Get Config File Path.vi"("error in (no error)"=w153) -> ("XML File Path"=w237:path)  [unwired: 9 in, 1 out]
            n90 = control-ref of="Montages"() -> (w164:refnum<vi>)
            n91 = Bundle By Name(cluster=w163, "Settings.Montage selection.Montages Ref"=w164, "Settings.Log File Base Path"=w149) -> (w162:T6)
            n92 = Format Into String(format string="Settings file located at: \"%s\"", w237) -> (resulting string=w236:string)  [unwired: 2 in, 1 out]
            n93 = Index Array(array=w233, index #1=0 ("index")) -> (element #1=w232:T19, element #2=w224:T19, element #3=w223:T19, element #4=w222:T19, element #5=w221:T19, element #6=w220:T19, element #7=w219:T19, element #8=w218:T19, element #9=w217:T19, element #10=w216:T19, element #11=w215:T19, element #12=w214:T19, element #13=w213:T19, element #14=w212:T19, element #15=w211:T19, element #16=w210:T19)  [unwired: 15 in]
            n94 = call "Status Updated.vi"("Status"=w236) -> ()  [unwired: 10 in, 1 out]
            n95 = Unbundle By Name(w162) -> ("Settings.Montage selection.Montages Ref"=w165:refnum<vi>, "Settings.Montage selection.Selected Montage Number"=w160:u8, "Settings Tab"=w156:refnum<vi>)
            n96 = Unbundle By Name(w232) -> ("Channel Name"=w231:string, "Channel Enabled"=w230:bool, "Channel Referenced"=w229:bool)
            n97 = Unbundle By Name(w224) -> ("Channel Name"=w227:string, "Channel Enabled"=w226:bool, "Channel Referenced"=w225:bool)
            n98 = Unbundle By Name(w223) -> ("Channel Name"=w209:string, "Channel Enabled"=w208:bool, "Channel Referenced"=w207:bool)
            n99 = Unbundle By Name(w222) -> ("Channel Name"=w206:string, "Channel Enabled"=w205:bool, "Channel Referenced"=w204:bool)
            n100 = Unbundle By Name(w221) -> ("Channel Name"=w203:string, "Channel Enabled"=w202:bool, "Channel Referenced"=w201:bool)
            n101 = Unbundle By Name(w220) -> ("Channel Name"=w200:string, "Channel Enabled"=w199:bool, "Channel Referenced"=w198:bool)
            n102 = Unbundle By Name(w219) -> ("Channel Name"=w197:string, "Channel Enabled"=w196:bool, "Channel Referenced"=w195:bool)
            n103 = Unbundle By Name(w218) -> ("Channel Name"=w194:string, "Channel Enabled"=w193:bool, "Channel Referenced"=w192:bool)
            n104 = Unbundle By Name(w217) -> ("Channel Name"=w191:string, "Channel Enabled"=w190:bool, "Channel Referenced"=w189:bool)
            n105 = Unbundle By Name(w216) -> ("Channel Name"=w188:string, "Channel Enabled"=w187:bool, "Channel Referenced"=w186:bool)
            n106 = Unbundle By Name(w215) -> ("Channel Name"=w185:string, "Channel Enabled"=w184:bool, "Channel Referenced"=w183:bool)
            n107 = Unbundle By Name(w214) -> ("Channel Name"=w182:string, "Channel Enabled"=w181:bool, "Channel Referenced"=w180:bool)
            n108 = Unbundle By Name(w213) -> ("Channel Name"=w179:string, "Channel Enabled"=w178:bool, "Channel Referenced"=w177:bool)
            n109 = Unbundle By Name(w212) -> ("Channel Name"=w176:string, "Channel Enabled"=w175:bool, "Channel Referenced"=w174:bool)
            n110 = Unbundle By Name(w211) -> ("Channel Name"=w173:string, "Channel Enabled"=w172:bool, "Channel Referenced"=w171:bool)
            n111 = Unbundle By Name(w210) -> ("Channel Name"=w170:string, "Channel Enabled"=w169:bool, "Channel Referenced"=w168:bool)
            n112 = property class="TabCtl (strict)"(reference=w156, "Value"=enum32{"Main", "Montage Adder"}."Main") -> ()  [unwired: 1 in, 2 out]
            n113 = call "Get all Channel Settings File Names.vi"() -> ("Channel Settings Files"=w161:string[])  [unwired: 11 in]
            n114 = local write "Ref ch 19"(w208) -> ()
            n115 = local write "Name Ch 17"(w231) -> ()
            n116 = local write "En ch 17"(w230) -> ()
            n117 = local write "Ref ch 17"(w229) -> ()
            n118 = local write "Name Ch 18"(w227) -> ()
            n119 = local write "En ch 18"(w226) -> ()
            n120 = local write "Ref ch 18"(w225) -> ()
            n121 = local write "Name Ch 19"(w209) -> ()
            n122 = local write "Name Ch 20"(w206) -> ()
            n123 = local write "En ch 20"(w205) -> ()
            n124 = local write "Ref ch 20"(w204) -> ()
            n125 = local write "Name Ch 21"(w203) -> ()
            n126 = local write "En ch 21"(w202) -> ()
            n127 = local write "Ref ch 21"(w201) -> ()
            n128 = local write "Name Ch 22"(w200) -> ()
            n129 = local write "En ch 22"(w199) -> ()
            n130 = local write "Ref ch 22"(w198) -> ()
            n131 = local write "Name Ch 23"(w197) -> ()
            n132 = local write "En ch 23"(w196) -> ()
            n133 = local write "Ref ch 23"(w195) -> ()
            n134 = local write "Name Ch 24"(w194) -> ()
            n135 = local write "En ch 24"(w193) -> ()
            n136 = local write "Ref ch 24"(w192) -> ()
            n137 = local write "Name Ch 25"(w191) -> ()
            n138 = local write "En ch 25"(w190) -> ()
            n139 = local write "Ref ch 25"(w189) -> ()
            n140 = Bundle By Name(cluster=w162, "Settings.Montage selection.Montages Names"=w161) -> (w145:T6)
            n141 = local write "Ref ch 3"(w207) -> ()
            n142 = local write "Name Ch 26"(w188) -> ()
            n143 = local write "En ch 26"(w187) -> ()
            n144 = local write "Ref ch 26"(w186) -> ()
            n145 = local write "Name Ch 27"(w185) -> ()
            n146 = local write "En ch 27"(w184) -> ()
            n147 = local write "Ref ch 27"(w183) -> ()
            n148 = local write "Name Ch 28"(w182) -> ()
            n149 = local write "En ch 28"(w181) -> ()
            n150 = local write "Ref ch 28"(w180) -> ()
            n151 = local write "Name Ch 29"(w179) -> ()
            n152 = local write "En ch 29"(w178) -> ()
            n153 = local write "Ref ch 29"(w177) -> ()
            n154 = local write "Name Ch 30"(w176) -> ()
            n155 = local write "En ch 30"(w175) -> ()
            n156 = local write "Ref ch 30"(w174) -> ()
            n157 = local write "Name Ch 31"(w173) -> ()
            n158 = local write "En ch 31"(w172) -> ()
            n159 = local write "Ref ch 31"(w171) -> ()
            n160 = local write "Name Ch 32"(w170) -> ()
            n161 = local write "En ch 32"(w169) -> ()
            n162 = local write "Ref ch 32"(w168) -> ()
            n163 = property class="LstBox (strict)"(reference=w165, "Item Names"=w161, "Value"=w160) -> ()  [unwired: 1 in, 2 out]
            n164 = control-ref of="En ch 6"() -> (w138:refnum<vi>)
            n165 = control-ref of="En ch 7"() -> (w137:refnum<vi>)
            n166 = control-ref of="En ch 9"() -> (w135:refnum<vi>)
            n167 = control-ref of="En ch 4"() -> (w140:refnum<vi>)
            n168 = control-ref of="En ch 5"() -> (w139:refnum<vi>)
            n169 = control-ref of="En ch 8"() -> (w136:refnum<vi>)
            n170 = control-ref of="En ch 16"() -> (w128:refnum<vi>)
            n171 = control-ref of="En ch 1"() -> (w143:refnum<vi>)
            n172 = control-ref of="En ch 11"() -> (w133:refnum<vi>)
            n173 = control-ref of="Delete Montage"() -> (w127:refnum<vi>)
            n174 = control-ref of="En ch 2"() -> (w142:refnum<vi>)
            n175 = control-ref of="En ch 14"() -> (w130:refnum<vi>)
            n176 = control-ref of="En ch 15"() -> (w129:refnum<vi>)
            n177 = control-ref of="En ch 3"() -> (w141:refnum<vi>)
            n178 = control-ref of="En ch 10"() -> (w134:refnum<vi>)
            n179 = control-ref of="En ch 12"() -> (w132:refnum<vi>)
            n180 = control-ref of="En ch 13"() -> (w131:refnum<vi>)
            n181 = Bundle By Name(cluster=w145, "Controls UI.En ch 1"=w143, "Controls UI.En ch 2"=w142, "Controls UI.En ch 3"=w141, "Controls UI.En ch 4"=w140, "Controls UI.En ch 5"=w139, "Controls UI.En ch 6"=w138, "Controls UI.En ch 7"=w137, "Controls UI.En ch 8"=w136, "Controls UI.En ch 9"=w135, "Controls UI.En ch 10"=w134, "Controls UI.En ch 11"=w133, "Controls UI.En ch 12"=w132, "Controls UI.En ch 13"=w131, "Controls UI.En ch 14"=w130, "Controls UI.En ch 15"=w129, "Controls UI.En ch 16"=w128, "Controls UI.Delete Montage"=w127) -> (w144:T6)
          }
          frame "---Module Specific---" {
            # "Separator -- The following cases handle messages specific to this Module."
          }
          frame "Update Application Settings" {
            # "Request Settings Editor to return the latest settings. The Settings Editor can send the applications settings as a reply or via broadcast."
            n182 = Unbundle By Name(w265) -> ("Settings.EEG Channels"=w259:T1, "Settings.Signal Type"=w263:T4, "Settings.Calibration Array"=w262:T3[], "Settings.Log File Base Path"=w261:path, "Settings.Soft Trig enum"=w258:T2, "Settings.Montage selection"=w257:T20, "Settings.LSL En enum"=w256:enum16{"LSL Disabled", "LSL Enabled"})
            n183 = Variant To Data(error in=w271, type=T11 {"Wait Notifier"=refnum, "wait for reply"=FALSE} ("Update Application Settings Argument"), Variant=w270) -> (data=w268:T11, error out=w272:errorcluster)
            n184 = Bundle By Name(cluster=T16 {"Settings"={"Signal Type"=enum."Sine Wave", "Calibration Array"=[], "Log File Base Path"=path "", "EEG Channels"={"16 EEG Channels"=[], "Gain"=24}, "Soft Trig enum"=enum."Disable Soft Trigger", "Montage selection"={"Montages Ref"=refnum, "Selected Montage Number"=0, "Montages Names"=[]}, "LSL En enum"=enum."LSL Disabled"}, "error"={"status"=FALSE, "code"=0, "source"=""}} ("Update Application Settings (Reply Payload)"), "Settings.EEG Channels"=w259, "Settings.Signal Type"=w263, "Settings.Calibration Array"=w262, "Settings.Log File Base Path"=w261, "error"=w272, "Settings.Soft Trig enum"=w258, "Settings.Montage selection"=w257, "Settings.LSL En enum"=w256) -> (w260:T16)
            n185 = Unbundle By Name(w268) -> ("Wait Notifier"=w267:refnum<notifier>, "wait for reply"=w266:bool)
            n186 = case shown="True" w266 {
              tunnel: w267 -> [_ w274]
              tunnel: w260 -> [_ w273]
              frame False {
              }
              frame True {
                n187 = Send Notification(notification=w273, notifier=w274) -> ()  [unwired: 1 in, 2 out]
              }
            }
            n188 = call "Application Settings Updated.vi"("error in (no error)"=w272, "Reply Payload"=w260) -> ()  [unwired: 9 in, 1 out]
          }
          frame "Save Settings" {
            w373 = T19 {"Channel Name"="", "Channel No"=0, "Channel Enabled"=FALSE, "Channel Referenced"=FALSE} ("EEG Single Channel")
            # "The end user pressed OK button and the current values on the front panel are the new settings."
            n189 = control-ref of="This VI"() -> (w393:refnum<vi>)
            n190 = Unbundle By Name(w276) -> ("Settings.Montage selection.Montages Ref"=w275:refnum<vi>)
            n191 = call "Hide VI Panel.vi"("VI"=w393) -> ()  [unwired: 10 in, 1 out]
            n192 = call "Retrieve Selected Montage.vi"("input cluster"=w276) -> ("EEG Channels"=w343:T18)  [unwired: 9 in, 1 out]
            n193 = Index Array(array=w343, index #1=0 ("index")) -> (element #1=w342:T19, element #2=w332:T19, element #3=w331:T19, element #4=w330:T19, element #5=w326:T19, element #6=w322:T19, element #7=w321:T19, element #8=w320:T19, element #9=w319:T19, element #10=w318:T19, element #11=w302:T19, element #12=w301:T19, element #13=w300:T19, element #14=w299:T19, element #15=w298:T19, element #16=w297:T19)  [unwired: 15 in]
            n194 = Unbundle By Name(w297) -> ("Channel Name"=w281:string, "Channel Enabled"=w280:bool, "Channel Referenced"=w279:bool)
            n195 = Unbundle By Name(w299) -> ("Channel Name"=w287:string, "Channel Enabled"=w286:bool, "Channel Referenced"=w285:bool)
            n196 = Unbundle By Name(w298) -> ("Channel Name"=w284:string, "Channel Enabled"=w283:bool, "Channel Referenced"=w282:bool)
            n197 = Unbundle By Name(w318) -> ("Channel Name"=w305:string, "Channel Enabled"=w304:bool, "Channel Referenced"=w303:bool)
            n198 = Unbundle By Name(w302) -> ("Channel Name"=w296:string, "Channel Enabled"=w295:bool, "Channel Referenced"=w294:bool)
            n199 = Unbundle By Name(w301) -> ("Channel Name"=w293:string, "Channel Enabled"=w292:bool, "Channel Referenced"=w291:bool)
            n200 = Unbundle By Name(w300) -> ("Channel Name"=w290:string, "Channel Enabled"=w289:bool, "Channel Referenced"=w288:bool)
            n201 = Unbundle By Name(w320) -> ("Channel Name"=w311:string, "Channel Enabled"=w310:bool, "Channel Referenced"=w309:bool)
            n202 = Unbundle By Name(w319) -> ("Channel Name"=w308:string, "Channel Enabled"=w307:bool, "Channel Referenced"=w306:bool)
            n203 = Unbundle By Name(w326) -> ("Channel Name"=w325:string, "Channel Enabled"=w324:bool, "Channel Referenced"=w323:bool)
            n204 = Unbundle By Name(w322) -> ("Channel Name"=w317:string, "Channel Enabled"=w316:bool, "Channel Referenced"=w315:bool)
            n205 = Unbundle By Name(w321) -> ("Channel Name"=w314:string, "Channel Enabled"=w313:bool, "Channel Referenced"=w312:bool)
            n206 = Unbundle By Name(w331) -> ("Channel Name"=w335:string, "Channel Enabled"=w334:bool, "Channel Referenced"=w333:bool)
            n207 = Unbundle By Name(w330) -> ("Channel Name"=w329:string, "Channel Enabled"=w328:bool, "Channel Referenced"=w327:bool)
            n208 = Unbundle By Name(w342) -> ("Channel Name"=w341:string, "Channel Enabled"=w340:bool, "Channel Referenced"=w339:bool)
            n209 = Unbundle By Name(w332) -> ("Channel Name"=w338:string, "Channel Enabled"=w337:bool, "Channel Referenced"=w336:bool)
            n210 = Bundle(cluster=w373, "Channel Name"=w341, "Channel No"=u8 1, "Channel Enabled"=w340, "Channel Referenced"=w339) -> (w378:T19)
            n211 = Bundle(cluster=w373, "Channel Name"=w338, "Channel No"=u8 2, "Channel Enabled"=w337, "Channel Referenced"=w336) -> (w376:T19)
            n212 = Bundle(cluster=w373, "Channel Name"=w335, "Channel No"=u8 3, "Channel Enabled"=w334, "Channel Referenced"=w333) -> (w374:T19)
            n213 = Bundle(cluster=w373, "Channel Name"=w329, "Channel No"=u8 4, "Channel Enabled"=w328, "Channel Referenced"=w327) -> (w372:T19)
            n214 = Bundle(cluster=w373, "Channel Name"=w325, "Channel No"=u8 5, "Channel Enabled"=w324, "Channel Referenced"=w323) -> (w371:T19)
            n215 = Bundle(cluster=w373, "Channel Name"=w317, "Channel No"=u8 6, "Channel Enabled"=w316, "Channel Referenced"=w315) -> (w370:T19)
            n216 = Bundle(cluster=w373, "Channel Name"=w314, "Channel No"=u8 7, "Channel Enabled"=w313, "Channel Referenced"=w312) -> (w369:T19)
            n217 = Bundle(cluster=w373, "Channel Name"=w311, "Channel No"=u8 8, "Channel Enabled"=w310, "Channel Referenced"=w309) -> (w368:T19)
            n218 = Bundle(cluster=w373, "Channel Name"=w308, "Channel No"=u8 9, "Channel Enabled"=w307, "Channel Referenced"=w306) -> (w367:T19)
            n219 = Bundle(cluster=w373, "Channel Name"=w305, "Channel No"=u8 10, "Channel Enabled"=w304, "Channel Referenced"=w303) -> (w366:T19)
            n220 = Bundle(cluster=w373, "Channel Name"=w296, "Channel No"=u8 11, "Channel Enabled"=w295, "Channel Referenced"=w294) -> (w365:T19)
            n221 = Bundle(cluster=w373, "Channel Name"=w293, "Channel No"=u8 12, "Channel Enabled"=w292, "Channel Referenced"=w291) -> (w364:T19)
            n222 = Bundle(cluster=w373, "Channel Name"=w290, "Channel No"=u8 13, "Channel Enabled"=w289, "Channel Referenced"=w288) -> (w363:T19)
            n223 = Bundle(cluster=w373, "Channel Name"=w287, "Channel No"=u8 14, "Channel Enabled"=w286, "Channel Referenced"=w285) -> (w362:T19)
            n224 = Bundle(cluster=w373, "Channel Name"=w284, "Channel No"=u8 15, "Channel Enabled"=w283, "Channel Referenced"=w282) -> (w361:T19)
            n225 = Bundle(cluster=w373, "Channel Name"=w281, "Channel No"=u8 16, "Channel Enabled"=w280, "Channel Referenced"=w279) -> (w360:T19)
            n226 = Build Array(w378, w376, w374, w372, w371, w370, w369, w368, w367, w366, w365, w364, w363, w362, w361, w360) -> (w380:T18)
            n227 = property class="LstBox (strict)"(reference=w275) -> ("Value"=w278:i32)  [unwired: 1 in, 2 out]
            n228 = Bundle By Name(cluster="Settings.EEG Channels", "16 EEG Channels"=w380, "Gain"=u8 24) -> (w346:T1)
            n229 = Bundle By Name(cluster=w276, "Settings.Calibration Array"="Calibration Values", "Settings.Signal Type"="Signal Type", "Settings.Log File Base Path"="Log File Base Path", "Settings.EEG Channels"=w346, "Settings.Soft Trig enum"="Soft Trig enum", "Settings.Montage selection.Selected Montage Number"=w278, "Settings.LSL En enum"="LSL En enum") -> (w392:T6)
            n230 = Unbundle By Name(w392) -> ("Settings"=w387:T7)
            n231 = Bundle By Name(cluster=T16 {"Settings"={"Signal Type"=enum."Sine Wave", "Calibration Array"=[], "Log File Base Path"=path "", "EEG Channels"={"16 EEG Channels"=[], "Gain"=24}, "Soft Trig enum"=enum."Disable Soft Trigger", "Montage selection"={"Montages Ref"=refnum, "Selected Montage Number"=0, "Montages Names"=[]}, "LSL En enum"=enum."LSL Disabled"}, "error"={"status"=FALSE, "code"=0, "source"=""}} ("Reply Payload"), "Settings"=w387) -> (w388:T16)
            n232 = call "Save Settings to XML.vi"("Settings"=w387) -> ("error out"=w384:errorcluster)  [unwired: 10 in]
            n233 = call "Application Settings Updated.vi"("Reply Payload"=w388) -> ("error out"=w383:errorcluster)  [unwired: 10 in]
            n234 = Merge Errors(w385, w384, w383) -> (w386:errorcluster)
          }
          frame "Set CNV Montage" {
            w496 = T19 {"Channel Name"="", "Channel No"=0, "Channel Enabled"=FALSE, "Channel Referenced"=FALSE} ("EEG Single Channel")
            # "Set CNV Montage"
            n235 = Unbundle By Name(w468) -> ("Settings.Montage selection.Montages Ref"=w402:refnum<vi>)
            n236 = call "Retrieve CNV Montage.vi"("ListBox in"=w402) -> ("Valid?"=w399:bool, "Value"=w400:i32, "EEG Channels"=w401:T18)  [unwired: 8 in]
            n237 = Index Array(array=w401, index #1=0 ("index")) -> (element #1=w466:T19, element #2=w456:T19, element #3=w455:T19, element #4=w454:T19, element #5=w450:T19, element #6=w446:T19, element #7=w445:T19, element #8=w444:T19, element #9=w443:T19, element #10=w442:T19, element #11=w426:T19, element #12=w425:T19, element #13=w424:T19, element #14=w423:T19, element #15=w422:T19, element #16=w421:T19)  [unwired: 15 in]
            n238 = Unbundle By Name(w421) -> ("Channel Name"=w405:string, "Channel Enabled"=w404:bool, "Channel Referenced"=w403:bool)
            n239 = Unbundle By Name(w423) -> ("Channel Name"=w411:string, "Channel Enabled"=w410:bool, "Channel Referenced"=w409:bool)
            n240 = Unbundle By Name(w422) -> ("Channel Name"=w408:string, "Channel Enabled"=w407:bool, "Channel Referenced"=w406:bool)
            n241 = Unbundle By Name(w442) -> ("Channel Name"=w429:string, "Channel Enabled"=w428:bool, "Channel Referenced"=w427:bool)
            n242 = Unbundle By Name(w426) -> ("Channel Name"=w420:string, "Channel Enabled"=w419:bool, "Channel Referenced"=w418:bool)
            n243 = Unbundle By Name(w425) -> ("Channel Name"=w417:string, "Channel Enabled"=w416:bool, "Channel Referenced"=w415:bool)
            n244 = Unbundle By Name(w424) -> ("Channel Name"=w414:string, "Channel Enabled"=w413:bool, "Channel Referenced"=w412:bool)
            n245 = Unbundle By Name(w444) -> ("Channel Name"=w435:string, "Channel Enabled"=w434:bool, "Channel Referenced"=w433:bool)
            n246 = Unbundle By Name(w443) -> ("Channel Name"=w432:string, "Channel Enabled"=w431:bool, "Channel Referenced"=w430:bool)
            n247 = Unbundle By Name(w450) -> ("Channel Name"=w449:string, "Channel Enabled"=w448:bool, "Channel Referenced"=w447:bool)
            n248 = Unbundle By Name(w446) -> ("Channel Name"=w441:string, "Channel Enabled"=w440:bool, "Channel Referenced"=w439:bool)
            n249 = Unbundle By Name(w445) -> ("Channel Name"=w438:string, "Channel Enabled"=w437:bool, "Channel Referenced"=w436:bool)
            n250 = Unbundle By Name(w455) -> ("Channel Name"=w459:string, "Channel Enabled"=w458:bool, "Channel Referenced"=w457:bool)
            n251 = Unbundle By Name(w454) -> ("Channel Name"=w453:string, "Channel Enabled"=w452:bool, "Channel Referenced"=w451:bool)
            n252 = Unbundle By Name(w466) -> ("Channel Name"=w465:string, "Channel Enabled"=w464:bool, "Channel Referenced"=w463:bool)
            n253 = Unbundle By Name(w456) -> ("Channel Name"=w462:string, "Channel Enabled"=w461:bool, "Channel Referenced"=w460:bool)
            n254 = call-poly <vilib>:"Delacor_lib_QMH_Enqueue Message (poly).vi"("error in"=w396, "Message"="Update Montage", "Message Queue in"=w397) -> ("error out"=w395:errorcluster)  [unwired: 7 in, 1 out]
            n255 = Bundle(cluster=w496, "Channel Name"=w465, "Channel No"=u8 1, "Channel Enabled"=w464, "Channel Referenced"=w463) -> (w501:T19)
            n256 = Bundle(cluster=w496, "Channel Name"=w462, "Channel No"=u8 2, "Channel Enabled"=w461, "Channel Referenced"=w460) -> (w499:T19)
            n257 = Bundle(cluster=w496, "Channel Name"=w459, "Channel No"=u8 3, "Channel Enabled"=w458, "Channel Referenced"=w457) -> (w497:T19)
            n258 = Bundle(cluster=w496, "Channel Name"=w453, "Channel No"=u8 4, "Channel Enabled"=w452, "Channel Referenced"=w451) -> (w495:T19)
            n259 = Bundle(cluster=w496, "Channel Name"=w449, "Channel No"=u8 5, "Channel Enabled"=w448, "Channel Referenced"=w447) -> (w494:T19)
            n260 = Bundle(cluster=w496, "Channel Name"=w441, "Channel No"=u8 6, "Channel Enabled"=w440, "Channel Referenced"=w439) -> (w493:T19)
            n261 = Bundle(cluster=w496, "Channel Name"=w438, "Channel No"=u8 7, "Channel Enabled"=w437, "Channel Referenced"=w436) -> (w492:T19)
            n262 = Bundle(cluster=w496, "Channel Name"=w435, "Channel No"=u8 8, "Channel Enabled"=w434, "Channel Referenced"=w433) -> (w491:T19)
            n263 = Bundle(cluster=w496, "Channel Name"=w432, "Channel No"=u8 9, "Channel Enabled"=w431, "Channel Referenced"=w430) -> (w490:T19)
            n264 = Bundle(cluster=w496, "Channel Name"=w429, "Channel No"=u8 10, "Channel Enabled"=w428, "Channel Referenced"=w427) -> (w489:T19)
            n265 = Bundle(cluster=w496, "Channel Name"=w420, "Channel No"=u8 11, "Channel Enabled"=w419, "Channel Referenced"=w418) -> (w488:T19)
            n266 = Bundle(cluster=w496, "Channel Name"=w417, "Channel No"=u8 12, "Channel Enabled"=w416, "Channel Referenced"=w415) -> (w487:T19)
            n267 = Bundle(cluster=w496, "Channel Name"=w414, "Channel No"=u8 13, "Channel Enabled"=w413, "Channel Referenced"=w412) -> (w486:T19)
            n268 = Bundle(cluster=w496, "Channel Name"=w411, "Channel No"=u8 14, "Channel Enabled"=w410, "Channel Referenced"=w409) -> (w485:T19)
            n269 = Bundle(cluster=w496, "Channel Name"=w408, "Channel No"=u8 15, "Channel Enabled"=w407, "Channel Referenced"=w406) -> (w484:T19)
            n270 = Bundle(cluster=w496, "Channel Name"=w405, "Channel No"=u8 16, "Channel Enabled"=w404, "Channel Referenced"=w403) -> (w483:T19)
            n271 = Build Array(w501, w499, w497, w495, w494, w493, w492, w491, w490, w489, w488, w487, w486, w485, w484, w483) -> (w503:T18)
            n272 = Bundle By Name(cluster="Settings.EEG Channels 2", "16 EEG Channels"=w503, "Gain"=u8 24) -> (w469:T1)
            n273 = case shown="True" w399 {
              tunnel: [w513 w517] -> w512
              tunnel: w469 -> [_ w516]
              tunnel: w468 -> [w513 w515]
              tunnel: w400 -> [_ w514]
              frame False {
              }
              frame True {
                n274 = Bundle By Name(cluster=w515, "Settings.EEG Channels"=w516, "Settings.Montage selection.Selected Montage Number"=w514) -> (w517:T6)
              }
            }
            n275 = Unbundle By Name(w512) -> ("Settings"=w509:T7)
            n276 = Bundle By Name(cluster=T16 {"Settings"={"Signal Type"=enum."Sine Wave", "Calibration Array"=[], "Log File Base Path"=path "", "EEG Channels"={"16 EEG Channels"=[], "Gain"=24}, "Soft Trig enum"=enum."Disable Soft Trigger", "Montage selection"={"Montages Ref"=refnum, "Selected Montage Number"=0, "Montages Names"=[]}, "LSL En enum"=enum."LSL Disabled"}, "error"={"status"=FALSE, "code"=0, "source"=""}} ("Reply Payload"), "Settings"=w509) -> (w510:T16)
            n277 = call "Save Settings to XML.vi"("Settings"=w509) -> ("error out"=w507:errorcluster)  [unwired: 10 in]
            n278 = call "Application Settings Updated.vi"("Reply Payload"=w510) -> ("error out"=w506:errorcluster)  [unwired: 10 in]
            n279 = Merge Errors(w395, w507, w506) -> (w508:errorcluster)
          }
          frame "Set Eyes OC Montage" {
            w619 = T19 {"Channel Name"="", "Channel No"=0, "Channel Enabled"=FALSE, "Channel Referenced"=FALSE} ("EEG Single Channel")
            # "Set Eyes Open Close Montage"
            n280 = Unbundle By Name(w591) -> ("Settings.Montage selection.Montages Ref"=w525:refnum<vi>)
            n281 = call "Retrieve Eyes OC Montage.vi"("ListBox in"=w525) -> ("Valid?"=w522:bool, "Value"=w523:i32, "EEG Channels"=w524:T18)  [unwired: 8 in]
            n282 = Index Array(array=w524, index #1=0 ("index")) -> (element #1=w589:T19, element #2=w579:T19, element #3=w578:T19, element #4=w577:T19, element #5=w573:T19, element #6=w569:T19, element #7=w568:T19, element #8=w567:T19, element #9=w566:T19, element #10=w565:T19, element #11=w549:T19, element #12=w548:T19, element #13=w547:T19, element #14=w546:T19, element #15=w545:T19, element #16=w544:T19)  [unwired: 15 in]
            n283 = Unbundle By Name(w544) -> ("Channel Name"=w528:string, "Channel Enabled"=w527:bool, "Channel Referenced"=w526:bool)
            n284 = Unbundle By Name(w546) -> ("Channel Name"=w534:string, "Channel Enabled"=w533:bool, "Channel Referenced"=w532:bool)
            n285 = Unbundle By Name(w545) -> ("Channel Name"=w531:string, "Channel Enabled"=w530:bool, "Channel Referenced"=w529:bool)
            n286 = Unbundle By Name(w565) -> ("Channel Name"=w552:string, "Channel Enabled"=w551:bool, "Channel Referenced"=w550:bool)
            n287 = Unbundle By Name(w549) -> ("Channel Name"=w543:string, "Channel Enabled"=w542:bool, "Channel Referenced"=w541:bool)
            n288 = Unbundle By Name(w548) -> ("Channel Name"=w540:string, "Channel Enabled"=w539:bool, "Channel Referenced"=w538:bool)
            n289 = Unbundle By Name(w547) -> ("Channel Name"=w537:string, "Channel Enabled"=w536:bool, "Channel Referenced"=w535:bool)
            n290 = Unbundle By Name(w567) -> ("Channel Name"=w558:string, "Channel Enabled"=w557:bool, "Channel Referenced"=w556:bool)
            n291 = Unbundle By Name(w566) -> ("Channel Name"=w555:string, "Channel Enabled"=w554:bool, "Channel Referenced"=w553:bool)
            n292 = Unbundle By Name(w573) -> ("Channel Name"=w572:string, "Channel Enabled"=w571:bool, "Channel Referenced"=w570:bool)
            n293 = Unbundle By Name(w569) -> ("Channel Name"=w564:string, "Channel Enabled"=w563:bool, "Channel Referenced"=w562:bool)
            n294 = Unbundle By Name(w568) -> ("Channel Name"=w561:string, "Channel Enabled"=w560:bool, "Channel Referenced"=w559:bool)
            n295 = Unbundle By Name(w578) -> ("Channel Name"=w582:string, "Channel Enabled"=w581:bool, "Channel Referenced"=w580:bool)
            n296 = Unbundle By Name(w577) -> ("Channel Name"=w576:string, "Channel Enabled"=w575:bool, "Channel Referenced"=w574:bool)
            n297 = Unbundle By Name(w589) -> ("Channel Name"=w588:string, "Channel Enabled"=w587:bool, "Channel Referenced"=w586:bool)
            n298 = Unbundle By Name(w579) -> ("Channel Name"=w585:string, "Channel Enabled"=w584:bool, "Channel Referenced"=w583:bool)
            n299 = call-poly <vilib>:"Delacor_lib_QMH_Enqueue Message (poly).vi"("error in"=w519, "Message"="Update Montage", "Message Queue in"=w520) -> ("error out"=w518:errorcluster)  [unwired: 7 in, 1 out]
            n300 = Bundle(cluster=w619, "Channel Name"=w588, "Channel No"=u8 1, "Channel Enabled"=w587, "Channel Referenced"=w586) -> (w624:T19)
            n301 = Bundle(cluster=w619, "Channel Name"=w585, "Channel No"=u8 2, "Channel Enabled"=w584, "Channel Referenced"=w583) -> (w622:T19)
            n302 = Bundle(cluster=w619, "Channel Name"=w582, "Channel No"=u8 3, "Channel Enabled"=w581, "Channel Referenced"=w580) -> (w620:T19)
            n303 = Bundle(cluster=w619, "Channel Name"=w576, "Channel No"=u8 4, "Channel Enabled"=w575, "Channel Referenced"=w574) -> (w618:T19)
            n304 = Bundle(cluster=w619, "Channel Name"=w572, "Channel No"=u8 5, "Channel Enabled"=w571, "Channel Referenced"=w570) -> (w617:T19)
            n305 = Bundle(cluster=w619, "Channel Name"=w564, "Channel No"=u8 6, "Channel Enabled"=w563, "Channel Referenced"=w562) -> (w616:T19)
            n306 = Bundle(cluster=w619, "Channel Name"=w561, "Channel No"=u8 7, "Channel Enabled"=w560, "Channel Referenced"=w559) -> (w615:T19)
            n307 = Bundle(cluster=w619, "Channel Name"=w558, "Channel No"=u8 8, "Channel Enabled"=w557, "Channel Referenced"=w556) -> (w614:T19)
            n308 = Bundle(cluster=w619, "Channel Name"=w555, "Channel No"=u8 9, "Channel Enabled"=w554, "Channel Referenced"=w553) -> (w613:T19)
            n309 = Bundle(cluster=w619, "Channel Name"=w552, "Channel No"=u8 10, "Channel Enabled"=w551, "Channel Referenced"=w550) -> (w612:T19)
            n310 = Bundle(cluster=w619, "Channel Name"=w543, "Channel No"=u8 11, "Channel Enabled"=w542, "Channel Referenced"=w541) -> (w611:T19)
            n311 = Bundle(cluster=w619, "Channel Name"=w540, "Channel No"=u8 12, "Channel Enabled"=w539, "Channel Referenced"=w538) -> (w610:T19)
            n312 = Bundle(cluster=w619, "Channel Name"=w537, "Channel No"=u8 13, "Channel Enabled"=w536, "Channel Referenced"=w535) -> (w609:T19)
            n313 = Bundle(cluster=w619, "Channel Name"=w534, "Channel No"=u8 14, "Channel Enabled"=w533, "Channel Referenced"=w532) -> (w608:T19)
            n314 = Bundle(cluster=w619, "Channel Name"=w531, "Channel No"=u8 15, "Channel Enabled"=w530, "Channel Referenced"=w529) -> (w607:T19)
            n315 = Bundle(cluster=w619, "Channel Name"=w528, "Channel No"=u8 16, "Channel Enabled"=w527, "Channel Referenced"=w526) -> (w606:T19)
            n316 = Build Array(w624, w622, w620, w618, w617, w616, w615, w614, w613, w612, w611, w610, w609, w608, w607, w606) -> (w626:T18)
            n317 = Bundle By Name(cluster="Settings.EEG Channels 3", "16 EEG Channels"=w626, "Gain"=u8 24) -> (w592:T1)
            n318 = case shown="True" w522 {
              tunnel: [w636 w640] -> w635
              tunnel: w592 -> [_ w639]
              tunnel: w591 -> [w636 w638]
              tunnel: w523 -> [_ w637]
              frame False {
              }
              frame True {
                n319 = Bundle By Name(cluster=w638, "Settings.EEG Channels"=w639, "Settings.Montage selection.Selected Montage Number"=w637) -> (w640:T6)
              }
            }
            n320 = Unbundle By Name(w635) -> ("Settings"=w632:T7)
            n321 = Bundle By Name(cluster=T16 {"Settings"={"Signal Type"=enum."Sine Wave", "Calibration Array"=[], "Log File Base Path"=path "", "EEG Channels"={"16 EEG Channels"=[], "Gain"=24}, "Soft Trig enum"=enum."Disable Soft Trigger", "Montage selection"={"Montages Ref"=refnum, "Selected Montage Number"=0, "Montages Names"=[]}, "LSL En enum"=enum."LSL Disabled"}, "error"={"status"=FALSE, "code"=0, "source"=""}} ("Reply Payload"), "Settings"=w632) -> (w633:T16)
            n322 = call "Save Settings to XML.vi"("Settings"=w632) -> ("error out"=w630:errorcluster)  [unwired: 10 in]
            n323 = call "Application Settings Updated.vi"("Reply Payload"=w633) -> ("error out"=w629:errorcluster)  [unwired: 10 in]
            n324 = Merge Errors(w518, w630, w629) -> (w631:errorcluster)
          }
          frame "Restore Settings" {
            # "The end user pressed Cancel button, need to restore the current stored values for the controls on the front panel. No need to broadcast that the settings changed."
            n325 = Unbundle By Name(w646) -> ("Settings.Signal Type"=w645:T4, "Settings.Log File Base Path"=w644:path, "Settings.Soft Trig enum"=w642:T2, "Settings.LSL En enum"=w641:enum16{"LSL Disabled", "LSL Enabled"})  [unwired: 2 out]
            n326 = control-ref of="This VI"() -> (w643:refnum<vi>)
            n327 = call "Hide VI Panel.vi"("VI"=w643) -> ()  [unwired: 10 in, 1 out]
            n328 = local write "Signal Type"(w645) -> ()
            n329 = local write "Log File Base Path"(w644) -> ()
            n330 = local write "Soft Trig enum"(w642) -> ()
            n331 = local write "LSL En enum"(w641) -> ()
          }
          frame "---Copy This Frame---" {
            # "Duplicate this frame when creating new messages.  Change this comment in the duplicated frame to describe this message."
            n332 = Merge Errors(w650) -> (w649:errorcluster)
          }
          frame "Delete Selected Montage" {
            # "Delete selected Montage (Except Default)"
            n333 = invoke on="Delete Montage" class="Bool" method="Reinit To Default"(error in=w651) -> ()  [unwired: 2 in, 3 out]
            n334 = call "Delete Selected Montage.vi"("error in (no error)"=w651, "Data Cluster"=w659) -> ("error out"=w656:errorcluster)  [unwired: 8 in, 1 out]
            n335 = call-poly <vilib>:"Delacor_lib_QMH_Enqueue Message (poly).vi"("error in"=w656, "Message"="Update Montage List", "Message Queue in"=w657) -> ("error out"=w653:errorcluster, "Message Queue out"=w654:refnum<class "Delacor_lib_QMH_Message Queue.lvclass">)  [unwired: 7 in]
            n336 = call-poly <vilib>:"Delacor_lib_QMH_Enqueue Message (poly).vi"("error in"=w653, "Message"="Update Montage", "Message Queue in"=w654) -> ("error out"=w652:errorcluster)  [unwired: 7 in, 1 out]
          }
          frame "Enable all Ch settings" {
            # "Enable All Channels for selection in New Montage"
            n337 = Variant To Data(error in=w682, type=TRUE, Variant=w681) -> (data=w661:bool, error out=w660:errorcluster)
            n338 = Unbundle By Name(w679) -> ("Controls UI.En ch 1"=w678:refnum<vi>, "Controls UI.En ch 2"=w677:refnum<vi>, "Controls UI.En ch 3"=w676:refnum<vi>, "Controls UI.En ch 4"=w675:refnum<vi>, "Controls UI.En ch 5"=w674:refnum<vi>, "Controls UI.En ch 6"=w673:refnum<vi>, "Controls UI.En ch 7"=w672:refnum<vi>, "Controls UI.En ch 8"=w671:refnum<vi>, "Controls UI.En ch 9"=w670:refnum<vi>, "Controls UI.En ch 10"=w669:refnum<vi>, "Controls UI.En ch 11"=w668:refnum<vi>, "Controls UI.En ch 12"=w667:refnum<vi>, "Controls UI.En ch 13"=w666:refnum<vi>, "Controls UI.En ch 14"=w665:refnum<vi>, "Controls UI.En ch 15"=w664:refnum<vi>, "Controls UI.En ch 16"=w663:refnum<vi>)
            n339 = Build Array(w678, w677, w676, w675, w674, w673, w672, w671, w670, w669, w668, w667, w666, w665, w664, w663) -> (w662:refnum<vi>[])
            n340 = call "Update UI Control value.vi"("Boolean"=w661, "Array"=w662) -> ()  [unwired: 10 in]
          }
          frame "Update Montage List" {
            # "Update Montages for the List"
            n341 = Merge Errors(w690) -> (w689:errorcluster)
            n342 = Unbundle By Name(w683) -> ("Settings.Montage selection.Montages Ref"=w688:refnum<vi>, "Settings.Montage selection.Selected Montage Number"=w684:u8, "Settings Tab"=w686:refnum<vi>)
            n343 = property class="TabCtl (strict)"(reference=w686, "Value"=enum32{"Main", "Montage Adder"}."Main") -> ()  [unwired: 1 in, 2 out]
            n344 = call "Get all Channel Settings File Names.vi"() -> ("Channel Settings Files"=w687:string[])  [unwired: 11 in]
            n345 = Bundle By Name(cluster=w683, "Settings.Montage selection.Montages Names"=w687) -> ()  [unwired: 1 out]
            n346 = property class="LstBox (strict)"(reference=w688, "Item Names"=w687, "Value"=w684) -> ()  [unwired: 1 in, 2 out]
          }
          frame "Add Montage Tab" {
            # "Go to New Montage Tab"
            n347 = Merge Errors(w695) -> (w694:errorcluster)
            n348 = Unbundle By Name(w693) -> ("Settings Tab"=w691:refnum<vi>)
            n349 = property class="TabCtl (strict)"(reference=w691, "Value"=enum32{"Main", "Montage Adder"}."Montage Adder") -> ()  [unwired: 1 in, 2 out]
          }
          frame "Return Montage Tab" {
            # "Go to Main Settings Tab"
            n350 = Merge Errors(w700) -> (w699:errorcluster)
            n351 = Unbundle By Name(w698) -> ("Settings Tab"=w696:refnum<vi>)
            n352 = property class="TabCtl (strict)"(reference=w696, "Value"=enum32{"Main", "Montage Adder"}."Main") -> ()  [unwired: 1 in, 2 out]
          }
          frame "Add New Montage" {
            w717 = T19 {"Channel Name"="", "Channel No"=0, "Channel Enabled"=FALSE, "Channel Referenced"=FALSE} ("EEG Single Channel")
            # "Add New Montage"
            n353 = call-poly <vilib>:"Delacor_lib_QMH_Enqueue Message (poly).vi"("Message"="Update Montage List", "Message Queue in"=w702) -> ("error out"=w701:errorcluster)  [unwired: 8 in, 1 out]
            n354 = Bundle(cluster=w717, "Channel Name"="Name Ch 12", "Channel No"=u8 12, "Channel Enabled"="En ch 12", "Channel Referenced"="Ref ch 12") -> (w710:T19)
            n355 = Merge Errors(w791, w701) -> (w790:errorcluster)
            n356 = Bundle(cluster=w717, "Channel Name"="Name Ch 11", "Channel No"=u8 11, "Channel Enabled"="En ch 11", "Channel Referenced"="Ref ch 11") -> (w711:T19)
            n357 = Bundle(cluster=w717, "Channel Name"="Name Ch 10", "Channel No"=u8 10, "Channel Enabled"="En ch 10", "Channel Referenced"="Ref ch 10") -> (w712:T19)
            n358 = Bundle(cluster=w717, "Channel Name"="Name Ch 1", "Channel No"=u8 1, "Channel Enabled"="En ch 1", "Channel Referenced"="Ref ch 1") -> (w763:T19)
            n359 = Bundle(cluster=w717, "Channel Name"="Name Ch 2", "Channel No"=u8 2, "Channel Enabled"="En ch 2", "Channel Referenced"="Ref ch 2") -> (w762:T19)
            n360 = Bundle(cluster=w717, "Channel Name"="Name Ch 6", "Channel No"=u8 6, "Channel Enabled"="En ch 6", "Channel Referenced"="Ref ch 6") -> (w758:T19)
            n361 = Bundle(cluster=w717, "Channel Name"="Name Ch 5", "Channel No"=u8 5, "Channel Enabled"="En ch 5", "Channel Referenced"="Ref ch 5") -> (w759:T19)
            n362 = Bundle(cluster=w717, "Channel Name"="Name Ch 3", "Channel No"=u8 3, "Channel Enabled"="En ch 3", "Channel Referenced"="Ref ch 3") -> (w761:T19)
            n363 = Bundle(cluster=w717, "Channel Name"="Name Ch 4", "Channel No"=u8 4, "Channel Enabled"="En ch 4", "Channel Referenced"="Ref ch 4") -> (w760:T19)
            n364 = Bundle(cluster=w717, "Channel Name"="Name Ch 16", "Channel No"=u8 16, "Channel Enabled"="En ch 16", "Channel Referenced"="Ref ch 16") -> (w706:T19)
            n365 = Bundle(cluster=w717, "Channel Name"="Name Ch 15", "Channel No"=u8 15, "Channel Enabled"="En ch 15", "Channel Referenced"="Ref ch 15") -> (w707:T19)
            n366 = Bundle(cluster=w717, "Channel Name"="Name Ch 8", "Channel No"=u8 8, "Channel Enabled"="En ch 8", "Channel Referenced"="Ref ch 8") -> (w743:T19)
            n367 = Bundle(cluster=w717, "Channel Name"="Name Ch 7", "Channel No"=u8 7, "Channel Enabled"="En ch 7", "Channel Referenced"="Ref ch 7") -> (w744:T19)
            n368 = Bundle(cluster=w717, "Channel Name"="Name Ch 13", "Channel No"=u8 13, "Channel Enabled"="En ch 13", "Channel Referenced"="Ref ch 13") -> (w709:T19)
            n369 = Bundle(cluster=w717, "Channel Name"="Name Ch 14", "Channel No"=u8 14, "Channel Enabled"="En ch 14", "Channel Referenced"="Ref ch 14") -> (w708:T19)
            n370 = Bundle(cluster=w717, "Channel Name"="Name Ch 9", "Channel No"=u8 9, "Channel Enabled"="En ch 9", "Channel Referenced"="Ref ch 9") -> (w742:T19)
            n371 = Build Array(w763, w762, w761, w760, w759, w758, w744, w743, w742, w712, w711, w710, w709, w708, w707, w706) -> (w757:T18)
            n372 = Bundle By Name(cluster=T1 {"16 EEG Channels"=[], "Gain"=24} ("EEG Channels"), "16 EEG Channels"=w757) -> (w704:T1)
            n373 = call "Save New Channel Settings.vi"("New Montage Name"="New Montage Name", "EEG Channels"=w704) -> ()  [unwired: 10 in]
          }
          frame "Update Montage" {
            # "Display Selected Montage"
            n374 = call "Retrieve Selected Montage.vi"("input cluster"=w792) -> ("EEG Channels"=w841:T18)  [unwired: 9 in, 1 out]
            n375 = Index Array(array=w841, index #1=0 ("index")) -> (element #1=w858:T19, element #2=w856:T19, element #3=w855:T19, element #4=w854:T19, element #5=w853:T19, element #6=w852:T19, element #7=w851:T19, element #8=w850:T19, element #9=w849:T19, element #10=w848:T19, element #11=w847:T19, element #12=w846:T19, element #13=w845:T19, element #14=w844:T19, element #15=w843:T19, element #16=w842:T19)  [unwired: 15 in]
            n376 = Unbundle By Name(w858) -> ("Channel Name"=→"Name Ch 17":string, "Channel Enabled"=→"En ch 17":bool, "Channel Referenced"=→"Ref ch 17":bool)
            n377 = Unbundle By Name(w856) -> ("Channel Name"=→"Name Ch 18":string, "Channel Enabled"=→"En ch 18":bool, "Channel Referenced"=→"Ref ch 18":bool)
            n378 = Unbundle By Name(w855) -> ("Channel Name"=→"Name Ch 19":string, "Channel Enabled"=→"En ch 19":bool, "Channel Referenced"=→"Ref ch 19":bool)
            n379 = Unbundle By Name(w854) -> ("Channel Name"=→"Name Ch 20":string, "Channel Enabled"=→"En ch 20":bool, "Channel Referenced"=→"Ref ch 20":bool)
            n380 = Unbundle By Name(w853) -> ("Channel Name"=→"Name Ch 21":string, "Channel Enabled"=→"En ch 25":bool, "Channel Referenced"=→"Ref ch 21":bool)
            n381 = Unbundle By Name(w852) -> ("Channel Name"=→"Name Ch 22":string, "Channel Enabled"=→"En ch 26":bool, "Channel Referenced"=→"Ref ch 22":bool)
            n382 = Unbundle By Name(w851) -> ("Channel Name"=→"Name Ch 23":string, "Channel Enabled"=→"En ch 27":bool, "Channel Referenced"=→"Ref ch 23":bool)
            n383 = Unbundle By Name(w850) -> ("Channel Name"=→"Name Ch 24":string, "Channel Enabled"=→"En ch 28":bool, "Channel Referenced"=→"Ref ch 24":bool)
            n384 = Unbundle By Name(w849) -> ("Channel Name"=→"Name Ch 25":string, "Channel Enabled"=→"En ch 29":bool, "Channel Referenced"=→"Ref ch 25":bool)
            n385 = Unbundle By Name(w848) -> ("Channel Name"=→"Name Ch 26":string, "Channel Enabled"=→"En ch 30":bool, "Channel Referenced"=→"Ref ch 26":bool)
            n386 = Unbundle By Name(w847) -> ("Channel Name"=→"Name Ch 27":string, "Channel Enabled"=→"En ch 31":bool, "Channel Referenced"=→"Ref ch 27":bool)
            n387 = Unbundle By Name(w846) -> ("Channel Name"=→"Name Ch 28":string, "Channel Enabled"=→"En ch 32":bool, "Channel Referenced"=→"Ref ch 28":bool)
            n388 = Unbundle By Name(w845) -> ("Channel Name"=→"Name Ch 29":string, "Channel Enabled"=→"En ch 21":bool, "Channel Referenced"=→"Ref ch 29":bool)
            n389 = Unbundle By Name(w844) -> ("Channel Name"=→"Name Ch 30":string, "Channel Enabled"=→"En ch 22":bool, "Channel Referenced"=→"Ref ch 30":bool)
            n390 = Unbundle By Name(w843) -> ("Channel Name"=→"Name Ch 31":string, "Channel Enabled"=→"En ch 23":bool, "Channel Referenced"=→"Ref ch 31":bool)
            n391 = Unbundle By Name(w842) -> ("Channel Name"=→"Name Ch 32":string, "Channel Enabled"=→"En ch 24":bool, "Channel Referenced"=→"Ref ch 32":bool)
            n392 = Merge Errors(w860) -> (w859:errorcluster)
          }
          frame "---Exit and Error Handling---" {
            # "Separator - The following cases handle errors and exit messages."
          }
          frame "Error" {
            # "Error - Check the error message data and respond accordingly. This message is sent by the \"Error Handler\" VIs at the end of each loop in this application."
            n393 = property class="Module Admin"(reference=w864) -> ("Accessors:External Launch"=w863:bool)  [unwired: 1 in, 2 out]
            n394 = Variant To Data(error in=w872, type=errorcluster {"status"=FALSE, "code"=0, "source"=""} ("error constant"), Variant=w866) -> (data=w873:errorcluster, error out=w870:errorcluster)
            n395 = call "Error Reported.vi"("Error"=w873) -> ()  [unwired: 10 in, 1 out]
            n396 = case shown="False" w863 {
              tunnel: [w878 _] -> w869
              tunnel: w865 -> [w876 _]
              tunnel: w873 -> [w877 _]
              frame False {
                # "If the module is running standalone, then pop up an error dialog and call the \"Exit\" message."
                n397 = call <vilib>:"Simple Error Handler.vi"("error in (no error)"=w877) -> ()  [unwired: 4 in, 5 out]
                n398 = call-poly <vilib>:"Delacor_lib_QMH_Enqueue Message (poly).vi"("Priority Message? (F)"=TRUE, "Message"="Exit", "Message Queue in"=w876) -> ("error out"=w878:errorcluster)  [unwired: 7 in, 1 out]
              }
              frame True {
                # "If the module was launched externally, calling the Error Reported broadcast VI is the only action performed by the \"Error\" message. The module's caller can then process the error appropriately."
              }
            }
            n399 = Merge Errors(w870, w869) -> (w868:errorcluster)
            n400 = local write "error out"(w868) -> ()
          }
          frame "Exit" {
            w883 = 91  # 91: not all Exit messages will have an argument
            w885 = TRUE  # Stop the VI
            # "Release the message queue reference"
            # "Exit - Exit the application."
            n401 = Variant To Data(error in=w893, type=T10 {"Origin"="", "Exit via Stop Module Req?"=FALSE, "Wait for Module to stop?"=FALSE} ("Stop Argument"), Variant=w884) -> (data=w881:T10, error out=w889:errorcluster)
            n402 = call <vilib>:"Clear Errors.vi"("error in (no error)"=w889, "specific error code to clear (0: all)"=w883) -> ("error out"=w892:errorcluster)  [unwired: 4 in, 1 out]
            n403 = call-dynamic "Delacor_lib_QMH_Release Message Queue.vi"("error in"=w892, "Message Queue"=w887) -> ("error out"=w891:errorcluster)  [unwired: 9 in]
            n404 = control-ref of="This VI"() -> (w880:refnum<vi>)
            n405 = call "Handle Exit.vi"("Stop Argument"=w881, "Admin in"=w879, "VI reference"=w880) -> ("error out"=w888:errorcluster)  [unwired: 7 in, 1 out]
            n406 = Merge Errors(w891, w888) -> (w890:errorcluster)
            n407 = call "Error Reported.vi"("Error"=w890) -> ()  [unwired: 10 in, 1 out]
          }
          frame Default {
            # "'Default' case only runs if there is a message that isn't defined in any of the other cases.  Output a programming error."
            n408 = call "Module Name--constant.vi"() -> ("Module Name"=w894:string)  [unwired: 11 in]
            n409 = xnode "Error Ring"("parameter 0"=w895, "parameter 1"=w894) -> ("error out"=w899:errorcluster)
            n410 = Merge Errors(w897, w899) -> (w898:errorcluster)
          }
        }
        n411 = call-dynamic "Delacor_lib_QMH_Error Handler - Message Handling Loop.vi"("error in"=w126, "Message Queue in"=w117) -> ("dup error in"=w123:errorcluster)  [unwired: 8 in, 1 out]
      }
    }
    frame Error {
      # "Synchronize Caller Events.vi will inform Start Module.vi that the module has launched and will let the code calling Start Module.vi register for broadcasts and would permit the caller receive the broadcast that an error occurred at launch time."
      n412 = call "Synchronize Caller Events.vi"("Singleton Module Admin in"=w911) -> ("error out"=w916:errorcluster)  [unwired: 9 in, 1 out]
      n413 = call-dynamic "Delacor_lib_QMH_Release Message Queue.vi"("error in"=w909, "Message Queue"=w910) -> ("error out"=w908:errorcluster)  [unwired: 9 in]
      n414 = call "Module Name--constant.vi"() -> ("Module Name"=w914:string)  [unwired: 11 in]
      n415 = Merge Errors(w908, w916) -> (w917:errorcluster)
      n416 = Format Into String(format string="An error occurred during initialization. %s is no longer running.", w914) -> (resulting string=w912:string)  [unwired: 2 in, 1 out]
      n417 = call "Error Reported.vi"("Additional Information"=w912, "Error"=w917) -> ()  [unwired: 9 in, 1 out]
    }
  }
  n418 = Merge Errors(w14, w17) -> (w13:errorcluster)
  n419 = call "Close Module.vi"("error in (no error)"=w13, "Module Admin in"=w8) -> ("error out"=w15:errorcluster, "External Launch"=w1:bool, "Module Admin out"=w2:refnum<class "Delacor_lib_QMH_Module Admin.lvclass">)  [unwired: 7 in]
  n420 = local write "Module Admin"(w2) -> ()
  n421 = Unregister For Events(event registration refnum=w7, error in=w15) -> (error out=w12:errorcluster)
  "error out" <- w12
  n422 = case "External Launch?" shown="True" w1 {
    tunnel: w12 -> [_ w918]
    frame False {
    }
    frame True {
      n423 = case shown="No Error" w918 {
        frame No Error {
          n424 = invoke class="VI" method="FP.Close"() -> ()  [unwired: 3 in, 3 out]
        }
        frame Error {
          n425 = invoke class="VI" method="FP.Open"("Activate"=TRUE ("Activate?")) -> ()  [unwired: 4 in, 5 out]
        }
      }
    }
  }
